vi "Oxford-VRM-v2-Main.vi"() -> ()   [LabVIEW 2016]
uses:
  <instrlib>/Mercury iXX/Public/Libraries/Magnet/Controls/Device (Read).ctl
  <instrlib>/Mercury iXX/Public/Controls/Manufacturing Data.ctl
  <instrlib>/Mercury iXX/Public/Libraries/Magnet/Controls/Signals (Read).ctl
  <instrlib>/Mercury iXX/Public/Controls/Unit String.ctl
  <instrlib>/Mercury iXX/Public/Libraries/Magnet/Controls/Identifier.ctl
  <instrlib>/Mercury iXX/Public/Libraries/Magnet/Controls/PSU Actions.ctl
  <instrlib>/Mercury iXX/Public/Controls/Mercury Reference.ctl
  <instrlib>/Mercury iXX/Public/Controls/Comms Transport Layer.ctl
  <instrlib>/Mercury iXX/Private/Controls/Query Dynamic Reference.ctl
  <vilib>/Analysis/coordinate.llb/3D Coordinate Conversion (Scalar).vi
  <instrlib>/Mercury iXX/Public/Libraries/Magnet/Open/Open Magnet Device.vi
  <instrlib>/Mercury iXX/Public/Libraries/Magnet/Configuration/Set/PSU Action Status (Set).vi
  <instrlib>/Mercury iXX/Public/Libraries/Magnet/Signals/Set/Target Field (Set).vi
  <instrlib>/Mercury iXX/Public/Libraries/Magnet/Signals/Set/Target Field Rate (Set).vi
  <userlib>/_OpenG.lib/error/error.llb/Filter Error Codes (Array)__ogtk.vi
  <instrlib>/Mercury iXX/Public/Libraries/System/Open/Open System.vi
  <instrlib>/Mercury iXX/Public/Libraries/System/Read/Catalogue (Read).vi
  <instrlib>/Mercury iXX/Public/Libraries/System/Read/Display Automatic Dimming (Read).vi
  <instrlib>/Mercury iXX/Public/Libraries/System/Read/Display Automatic Dimming Time (Read).vi
  <instrlib>/Mercury iXX/Public/Libraries/System/Read/Display Brightness (Read).vi
  <instrlib>/Mercury iXX/Public/Libraries/System/Read/Date (Read).vi
  <instrlib>/Mercury iXX/Public/Libraries/System/Read/Time (Read).vi
  <instrlib>/Mercury iXX/Public/Libraries/System/Read/DateTime (Read).vi
  <instrlib>/Mercury iXX/Public/Libraries/System/Read/HVer (Read).vi
  <instrlib>/Mercury iXX/Public/Libraries/System/Read/FVer (Read).vi
  <instrlib>/Mercury iXX/Public/Libraries/System/Read/Serial Number (Read).vi
  <instrlib>/Mercury iXX/Public/Libraries/System/Read/Flash Space (Read).vi
  <instrlib>/Mercury iXX/Public/Libraries/System/Read/Mode (Read).vi
  <instrlib>/Mercury iXX/Public/Libraries/System/Set/DateTime (Set).vi
  <instrlib>/Mercury iXX/Public/Libraries/Magnet/Configuration/Read/Magnet Device (Read).vi
  <instrlib>/Mercury iXX/Public/Libraries/Magnet/Configuration/Read/Serial Number (Read).vi
  <instrlib>/Mercury iXX/Public/Libraries/Magnet/Configuration/Read/Bipolar Output (Read).vi
  <instrlib>/Mercury iXX/Public/Libraries/Magnet/Configuration/Read/Output Configuration (Read).vi
  <instrlib>/Mercury iXX/Public/Libraries/Magnet/Configuration/Read/Current Limit (Read).vi
  <instrlib>/Mercury iXX/Public/Libraries/Magnet/Configuration/Read/Current to Field Factor (Read).vi
  <instrlib>/Mercury iXX/Public/Libraries/Magnet/Configuration/Read/Switch Present (Read).vi
  <instrlib>/Mercury iXX/Public/Libraries/Magnet/Configuration/Read/Software Voltage Limit (Read).vi
  <instrlib>/Mercury iXX/Public/Libraries/Magnet/Signals/Read/Current Rate (Read).vi
  <instrlib>/Mercury iXX/Public/Libraries/Magnet/Configuration/Read/PSU Action Status (Read).vi
  <instrlib>/Mercury iXX/Public/Libraries/Magnet/Signals/Read/Target Field (Read).vi
  <instrlib>/Mercury iXX/Public/Libraries/Magnet/Signals/Read/Field (Read).vi
  <instrlib>/Mercury iXX/Public/Libraries/Magnet/Signals/Read/Target Field Rate (Read).vi
  <instrlib>/Mercury iXX/Public/Libraries/Magnet/Signals/Read/Current (Read).vi
  <instrlib>/Mercury iXX/Public/Libraries/Magnet/Signals/Read/Voltage (Read).vi
  <instrlib>/Mercury iXX/Public/Libraries/Magnet/Configuration/Read/FVer (Read).vi
  <instrlib>/Mercury iXX/Mercury iXX.lvlib
  <instrlib>/Mercury iXX/Public/Libraries/System.lvlib
  <instrlib>/Mercury iXX/Public/Libraries/Magnet.lvlib
  <vilib>/Analysis/NI_AALPro.lvlib
panel:
  out "Firmware Version 2":string
  in  "Device Identifier 2":T1="GRPZ"
  in  "Tab Control":T2(tab)
  out "Z Magnet Status":string="Holding"
  out "Y Magnet Status":string="Holding"
  in  "Tab Control 3":enum32{"Main", "Zero/Clamp"}(tab)
  out "Time (min)":dbl
  in  "OK":bool
  in  "Remote Mode":bool
  in  "Hold":bool
  in  "To Set":bool
  in  "Send to IPS":bool
  in  "Sweep Rate (T/min)":dbl
  in  "Clamp":bool
  in  "To Zero":bool
  in  "Tab Control 2":enum32{"Cartesian", "Spherical"}(tab)
  in  "X Setpoint (T)":dbl
  in  "Y Setpoint (T)":dbl
  in  "Z Setpoint (T)":dbl
  out "X Target (T)":dbl
  out "X Field (T)":dbl=-0.0
  out "Y Target (T)":dbl
  out "Y Field (T)":dbl
  out "Z Target (T)":dbl
  out "Z Field (T)":dbl
  in  "R Setpoint (T)":dbl
  in  "Theta Setpoint (deg)":dbl
  in  "Phi Setpoint (deg)":dbl
  out "R Target (T)":dbl
  out "R Field (T)":dbl
  out "Theta Target (deg)":dbl
  out "Theta Field (deg)":dbl=180.0
  out "Phi Target (deg)":dbl
  out "Phi Field (deg)":dbl
  out "Sentinel":bool=TRUE
  out "Z Voltage (V)":dbl=-0.0001
  out "Z Current (A)":dbl
  out "Z Rate (T/min)":dbl=0.05
  out "Y Voltage (V)":dbl
  out "Y Current (A)":dbl=0.0001
  out "Y Rate (T/min)":dbl=0.0002
  out "X Voltage (V)":dbl=0.0003
  out "X Current (A)":dbl=-0.0001
  out "X Rate (T/min)":dbl=0.0002
  out "Magnet Response":string
  out "X Magnet Status":string="Holding"
  in  "Tab Control 4":enum32{"Graph", "Limits", "Definitions"}(tab)
  out "3D Graph":refnum<vi>(3d-picture)
  out "Legend":refnum<vi>(3d-picture)
  in  "Mercury Functions":enum32{"System: IPS", "Magnet"}(tab)
  out "time stamp":timestamp=timestamp(3548852719 s since 1904-01-01)
  out "Free Space 2":i32=167300 caption="Free Space (KB)"
  out "Set Date Response":string="VALID"
  out "String 2":string="NORM" caption="User Mode"
  out "Date":string="2016:06:15"
  out "Time":string="11:26:27"
  out "Hardware Version":string="65"
  out "Firmware Version":string="1.4.43"
  out "Serial Number":string="133350022"
  out "IPS Devices":string[](array[string])=["GRPX:PSU", "GRPY:PSU", "GRPZ:PSU", "MB1.T1:TEMP", "PSU.M1:PSU", "PSU.M2:PSU", "PSU.M3:PSU", "PSU.M4:PSU", "PSU.M5:PSU", "PSU.M6:PSU"]
  out "S/W Version(s)":string[](array[string])=["1.4.43\n"]
  out "Serial Number(s)":string[](array[string])=["65"]
  out "# of Instruments":i32=1
  out "Automatic Dimming":string="OFF"
  out "Dimming Time":string="3"
  out "Display Brightness":string="100"
  in  "IPS IP Address":string="130.49.180.67"
  out "Magnet Device Details":T3={"Manufacturing"={"Hardware Version"="NOT_FOUND", "Firmware Version"="NOT_FOUND", "Serial Number"="NOT_FOUND"}, "Nickname"="GRPX", "Bipolar Output"="ON", "String"="PARA", "Current Limit"=99.07, "AtoB"=49.5, "Inductance"=5.04, "Switch Present"="None", "Swh Htr Current"=100.0, "SW VLIM"=5.0, "V Trans Time"=0.0, "Magnet PSU Signals"={"Voltage"=0.0007, "Current"=0.0001, "Current Rate"=0.01, "Field"=0.0, "Field Rate"=0.0002, "Persistant Current"=0.0001, "Persistant Field"=0.0, "Target Current"=0.0, "Target Field"=0.0, "Target Current Rate"=0.01, "Target Field Rate"=0.0002, "Switch Heater Status (SWHT)"="ON", "Switch Heater Status (SWHN)"="ON"}, "PSU Action"="HOLD", "Status"="40000000", "Level Limit"=0.0, "Temperature Limit"=999.0} {"Temperature Limit" format="%#.1f"; "Level Limit" format="%#.1f"; "V Trans Time" format="%#.1f"; "SW VLIM" format="%#.1f"; "Swh Htr Current" format="%#.1f"; "Inductance" format="%#.1f"; "AtoB" format="%#.1f"; "Current Limit" format="%#.1f"}
  out "Mag S/N":string="NOT_FOUND"
  out "Bipolar Output":string="ON"
  out "Out Config":string="PARA" caption="Output Configuration"
  out "Current Limit":dbl=99.07 caption="Current Limit (A)" format="%#.1f"
  out "AtoB":dbl=49.5 caption="Current Field Factor (A/T)" format="%#.1f"
  out "Switch Present":string="None"
  out "SW VLIM":dbl=5.0 caption="Software Voltage Limit (V)" format="%#.1f"
  out "Unit 8":T6
  out "Unit 9":T6
  out "Unit 10":T6
  out "Current Rate":dbl=0.01
  out "PSU Act Stat":string="HOLD" caption="PSU Action Status"
  out "Unit 11":T6="A/min"
  in  "Device Identifier":T1="GRPX"
  out "Error List":T7(array[cluster])=[{"time"=timestamp(3548847490.5163774 s since 1904-01-01), "code"=-1950679035, "source"="Open Variable Connection in FGV_PSP - Mercury Remote.vi->Mercury iXX.lvlib:Oxford-VRM-v2-Main.vi"}, {"time"=timestamp(3548847496.0233774 s since 1904-01-01), "code"=-1950679035, "source"="Open Variable Connection in FGV_PSP - Mercury Remote.vi->Mercury iXX.lvlib:Oxford-VRM-v2-Main.vi"}, {"time"=timestamp(3548847520.519377 s since 1904-01-01), "code"=-1950679035, "source"="Open Variable Connection in FGV_PSP - Mercury Status.vi->Mercury iXX.lvlib:Oxford-VRM-v2-Main.vi"}, {"time"=timestamp(3548847557.480377 s since 1904-01-01), "code"=-1950679035, "source"="Open Variable Connection in FGV_PSP - Mercury Remote.vi->Mercury iXX.lvlib:Oxford-VRM-v2-Main.vi"}, {"time"=timestamp(3548847576.0283775 s since 1904-01-01), "code"=-1950679035, "source"="Open Variable Connection in FGV_PSP - Mercury Status.vi->Mercury iXX.lvlib:Oxford-VRM-v2-Main.vi"}]
  out "error out":errorcluster
  # "Oxford VRM v2 v2016/06/22"
  # "X \t\t\nCurrent (A)\tField (T)\t    Rate (T/min)\n0  - 30 \t   0    - 0.6 \t  0.06\n30 - 42\t    0.6  - 0.85\t  0.048\n42 - 60\t    0.85 - 1.2\t   0.042\n60 - 80\t    1.2  - 1.6\t   0.036\n80 - 99\t    1.6  - 2.0\t   0.024\n\nY \t\t\nCurrent (A)\tField (T)\t    Rate (T/min)\n0  - 30\t    0    - 0.6\t   0.048\n30 - 35\t    0.6  - 0.69\t  0.035\n35 - 45\t    0.69 - 0.89\t  0.03\n45 - 60\t    0.89 - 1.2\t   0.024\n60 - 80\t    1.2  - 1.58\t  0.018\n80 - 101\t   1.58 - 2\t     0.01\n\nZ \t\t\nCurrent (A)\tField (T)\t    Rate (T/min)\n0  - 30\t    0    - 2.6    0.26\n30 - 60\t    2.6  - 5.3\t   0.21\n60 - 80\t    5.3  - 7.1\t   0.16\n80 - 90\t    7.1  - 8\t     0.13\n90 - 101\t   8    - 9\t     0.1\n\n2 OR MORE AXES\n0.005 T/min"
  # "ITC: 101\nIPS: 102\nIPS VR: 67"
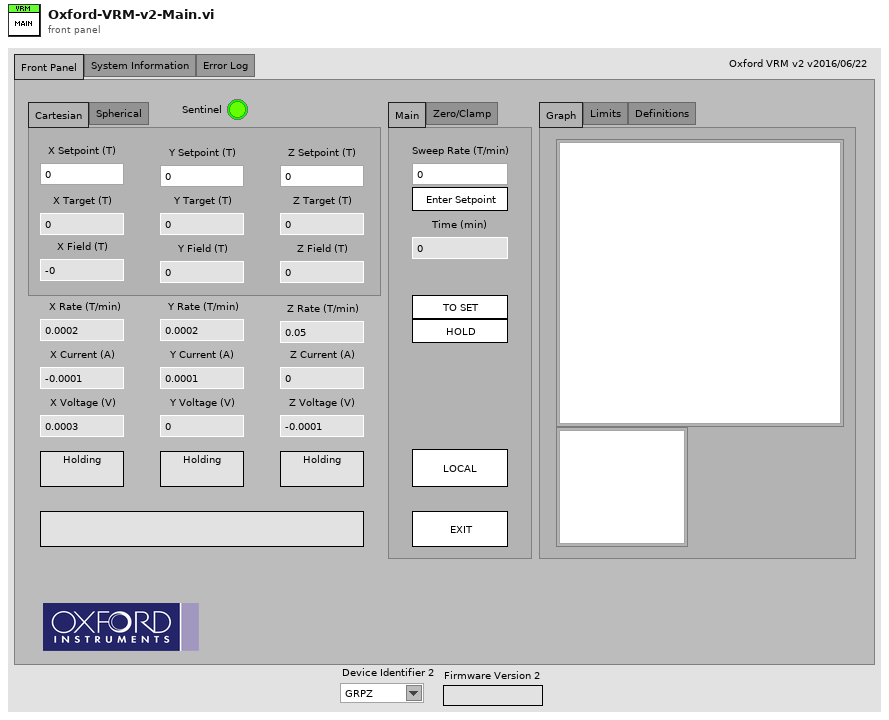
[diagram p1: front panel]
types:
  T1 = typedef "Mercury iXX.lvlib/Magnet.lvlib/Identifier.ctl" = string
  T2 = enum32{"Front Panel", "System Information", "Error Log"}
  T3 = typedef "Mercury iXX.lvlib/Magnet.lvlib/Device (Read).ctl" = cluster{"Manufacturing":T4, "Nickname":string, "Bipolar Output":string, "String":string, "Current Limit":dbl, "AtoB":dbl, "Inductance":dbl, "Switch Present":string, "Swh Htr Current":dbl, "SW VLIM":dbl, "V Trans Time":dbl, "Magnet PSU Signals":T5, "PSU Action":string, "Status":string, "Level Limit":dbl, "Temperature Limit":dbl}
  T4 = typedef "Mercury iXX.lvlib/Manufacturing Data.ctl" = cluster{"Hardware Version":string, "Firmware Version":string, "Serial Number":string}
  T5 = typedef "Mercury iXX.lvlib/Magnet.lvlib/Signals (Read).ctl" = cluster{"Voltage":dbl, "Current":dbl, "Current Rate":dbl, "Field":dbl, "Field Rate":dbl, "Persistant Current":dbl, "Persistant Field":dbl, "Target Current":dbl, "Target Field":dbl, "Target Current Rate":dbl, "Target Field Rate":dbl, "Switch Heater Status (SWHT)":string, "Switch Heater Status (SWHN)":string}
  T6 = typedef "Mercury iXX.lvlib/Unit String.ctl" = string
  T7 = cluster{"time":timestamp, "code":i32, "source":string}[]
  T8 = cluster{"Hold":bool, "Clamp":bool, "To Set":bool, "To Zero":bool, "Send to IPS":bool}
  T9 = cluster{"Bx0 (T)":dbl, "By0 (T)":dbl, "Bz0 (T)":dbl}
  T10 = cluster{"Bx (T)":dbl, "By (T)":dbl, "Bz (T)":dbl}
  T11 = enum32{"invalid app kind", "Development System", "Run Time System", "Student Edition", "Embedded LabVIEW", "Evaluation", "Custom"}
  T12 = cluster{"time":timestamp, "code":i32, "source":string}
  T13 = enum32{"Invalid", "Standard", "Closed", "Hidden", "Minimized", "Maximized"}
  T14 = typedef "Mercury iXX.lvlib/Comms Transport Layer.ctl" = enum16{"Ethernet TCP/IP", "USB", "ISOBus - RS-232", "GPIB"}
  T15 = cluster{"x action":string, "y action":string, "z action":string}
  T16 = typedef "Mercury iXX.lvlib/Mercury Reference.ctl" = cluster{"Comms":refnum<visa-resource-name>, "Device ID":string[], "Comms Layer":T14, "Command":string, "Query reference":T17}
  T17 = typedef "Mercury iXX.lvlib/Query Dynamic Reference.ctl" = refnum<vi>
  T18 = cluster{"Core":cluster{"Current VI Reference":refnum<vi>, "Close Panel on Exit?":bool}, "Mercury IPS Ref":T16, "sentinel":bool, "Error Log":cluster{"time":timestamp, "code":i32, "source":string}[]}
  T19 = cluster{"X Setpoint (T)":dbl, "Y Setpoint (T)":dbl, "Z Setpoint (T)":dbl, "Sweep Rate (T/min)":dbl}
  T20 = typedef "Mercury iXX.lvlib/Magnet.lvlib/PSU Actions.ctl" = string
  T21 = typedef "Mercury iXX.lvlib/Response String.ctl" = string
  T22 = cluster{"Rate_x (T/min)":dbl, "Rate_y (T/min)":dbl, "Rate_z (Tmin)":dbl}
  T23 = typedef "Filtered Error Details - Cluster__ogtk.ctl" = cluster{"code":i32, "source":string}
  T24 = cluster{"Current VI Reference":refnum<vi>, "Close Panel on Exit?":bool}
  T25 = typedef "Mercury iXX.lvlib/System.lvlib/User Mode.ctl" = string
  T26 = typedef "Mercury iXX.lvlib/Magnet.lvlib/Output Configuration.ctl" = string
  T27 = cluster{"X Target (T)":dbl, "Y Target (T)":dbl, "Z Target (T)":dbl, "X Field (T)":dbl, "Y Field (T)":dbl, "Z Field (T)":dbl, "X Rate (T/min)":dbl, "Y Rate (T/min)":dbl, "Z Rate (T/min)":dbl, "X Current (A)":dbl, "Y Current (A)":dbl, "Z Current (A)":dbl, "X Voltage (V)":dbl, "Y Voltage (V)":dbl, "Z Voltage (V)":dbl}
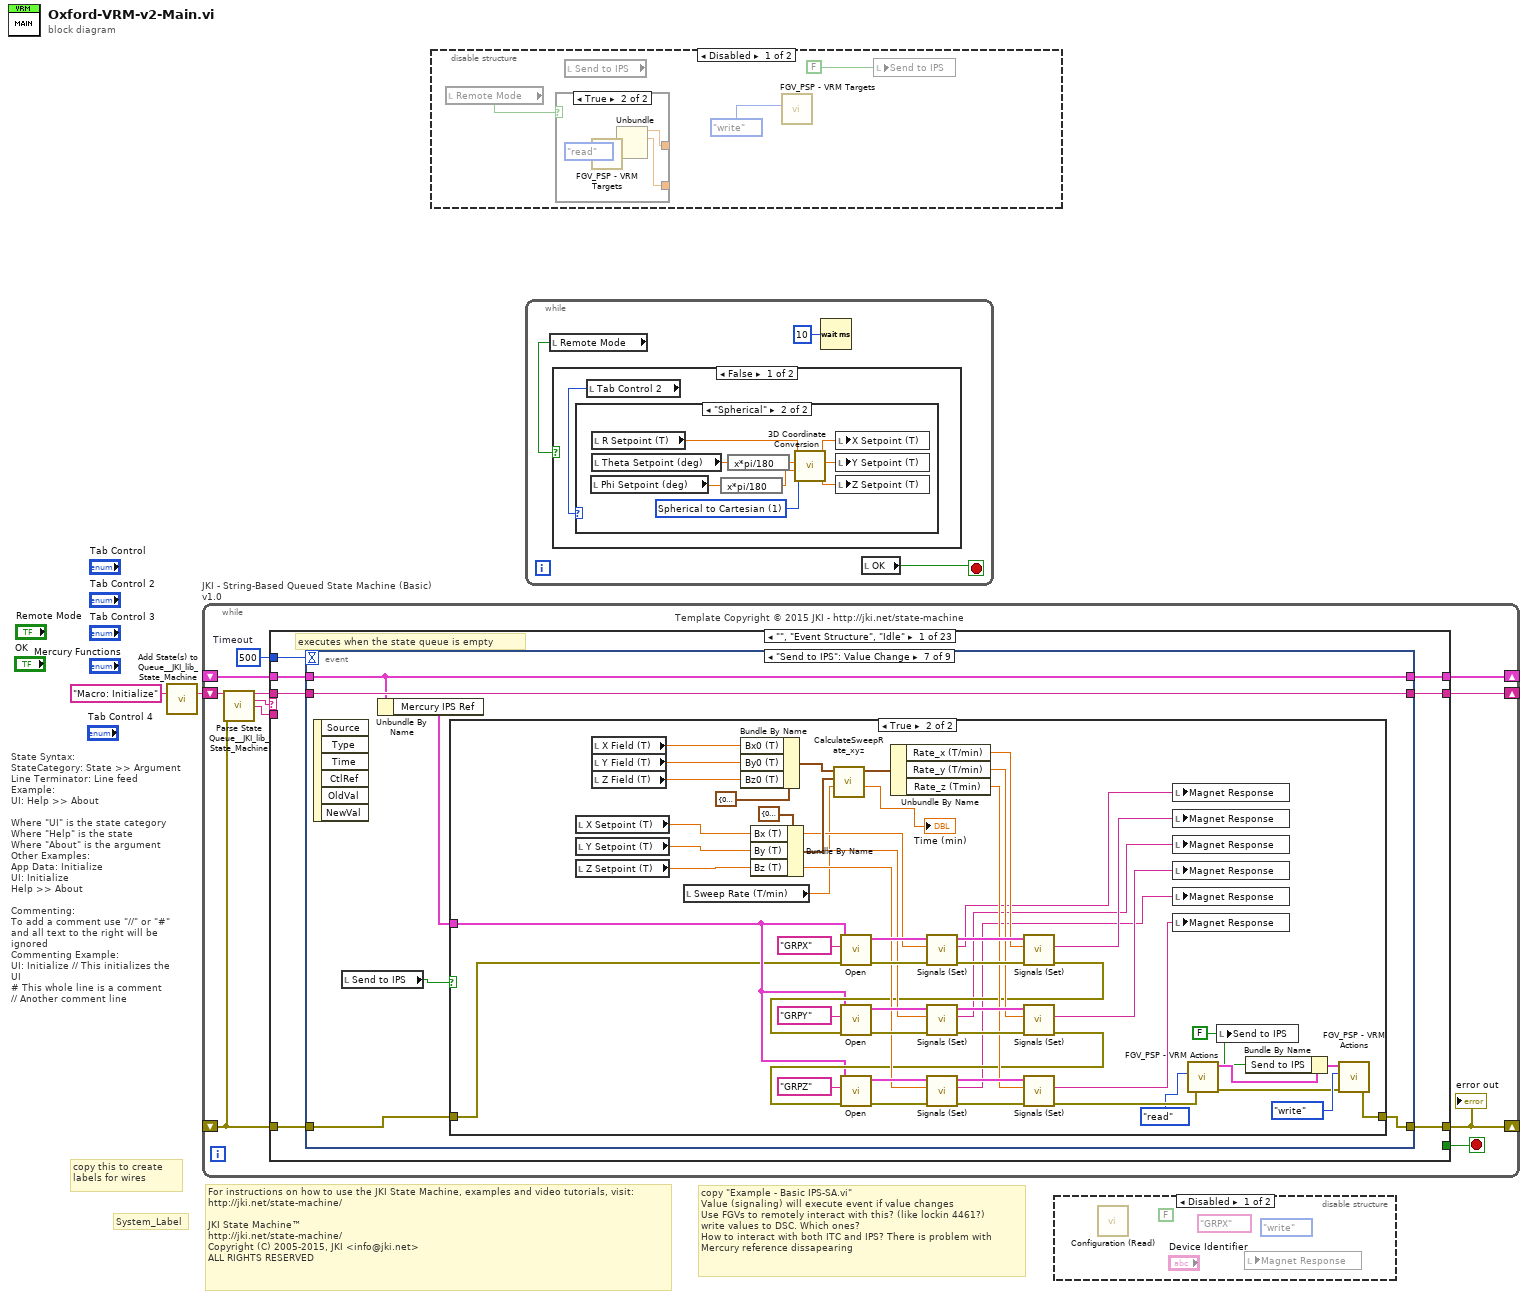
[diagram p0: block diagram]
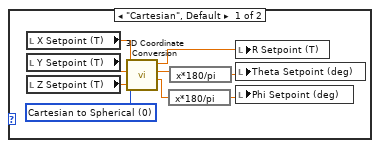
[diagram p2: hidden frame]
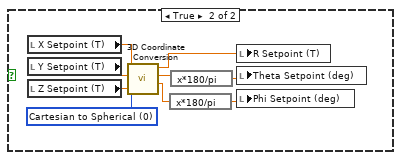
[diagram p3: hidden frame]
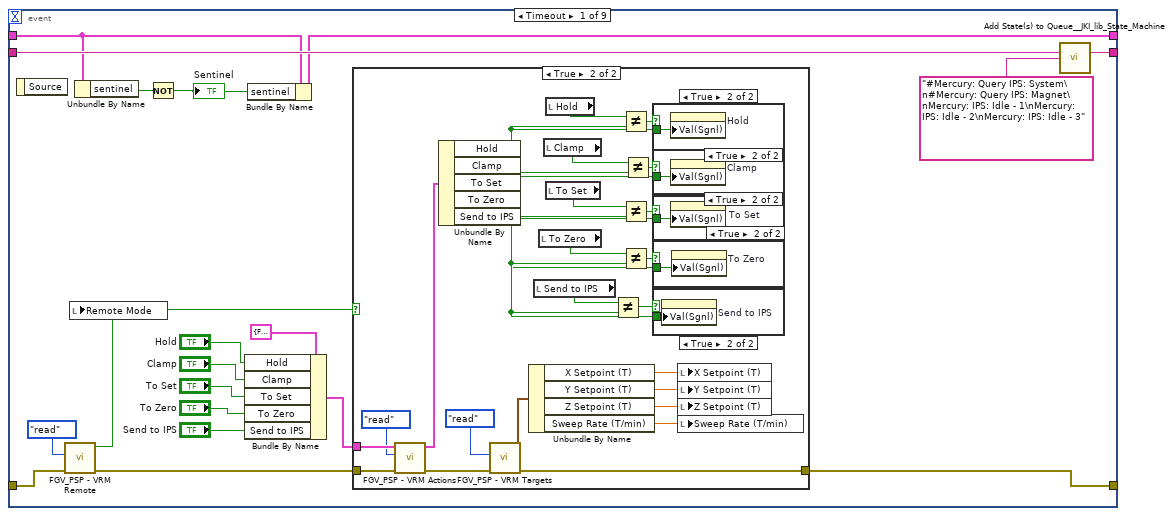
[diagram p7: hidden frame]
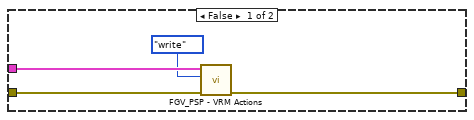
[diagram p8: hidden frame]
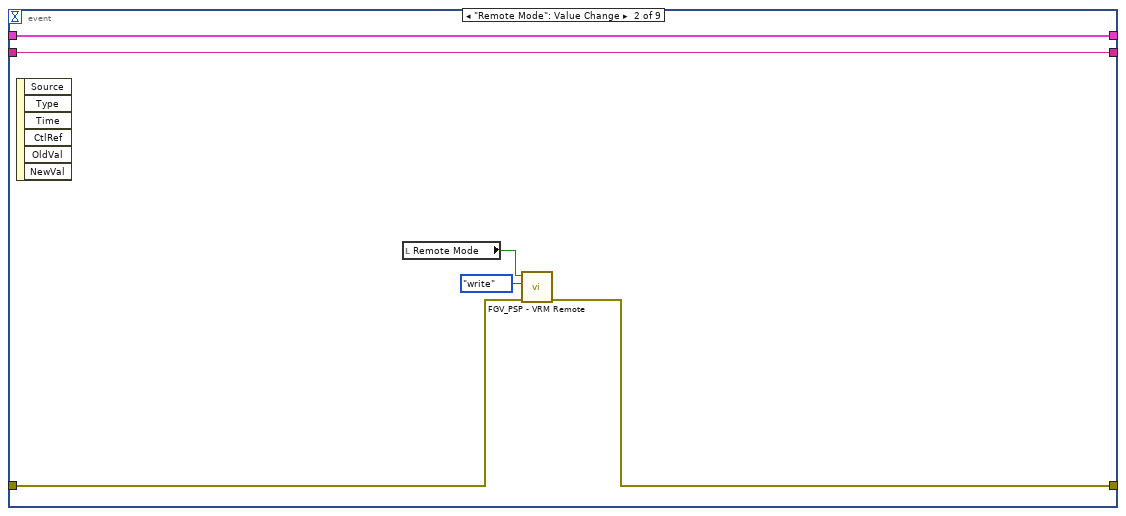
[diagram p14: hidden frame]
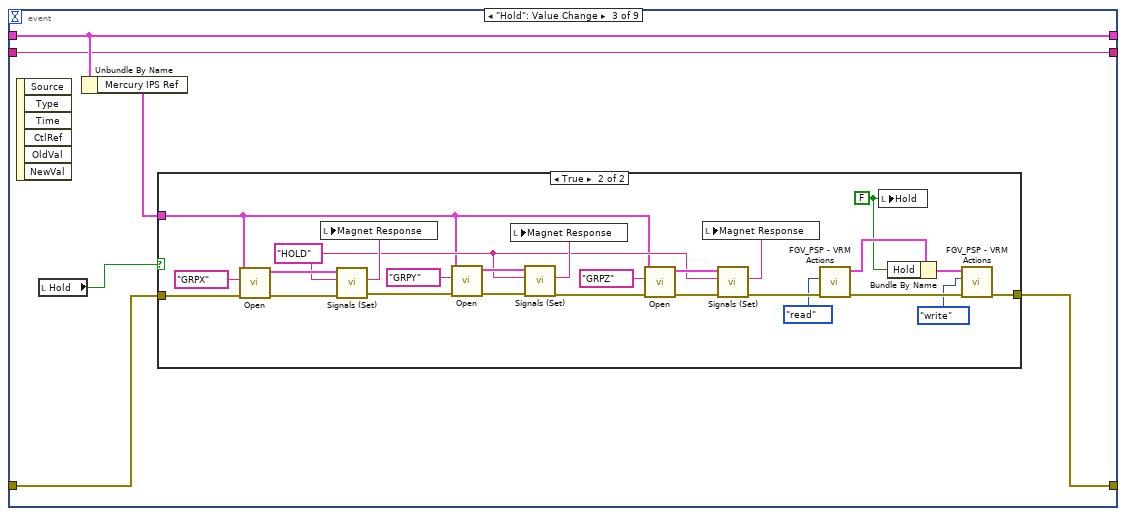
[diagram p15: hidden frame]
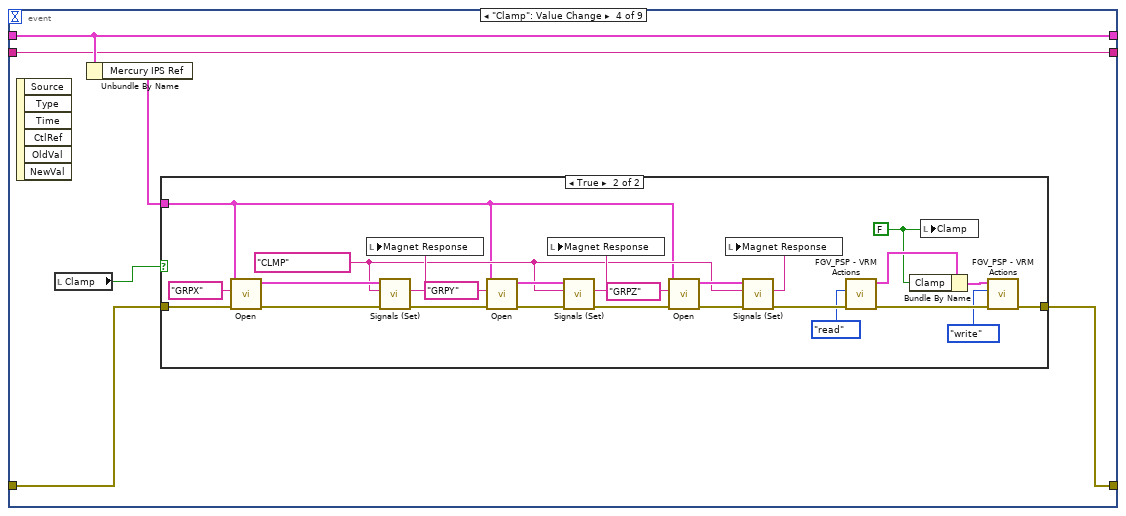
[diagram p17: hidden frame]
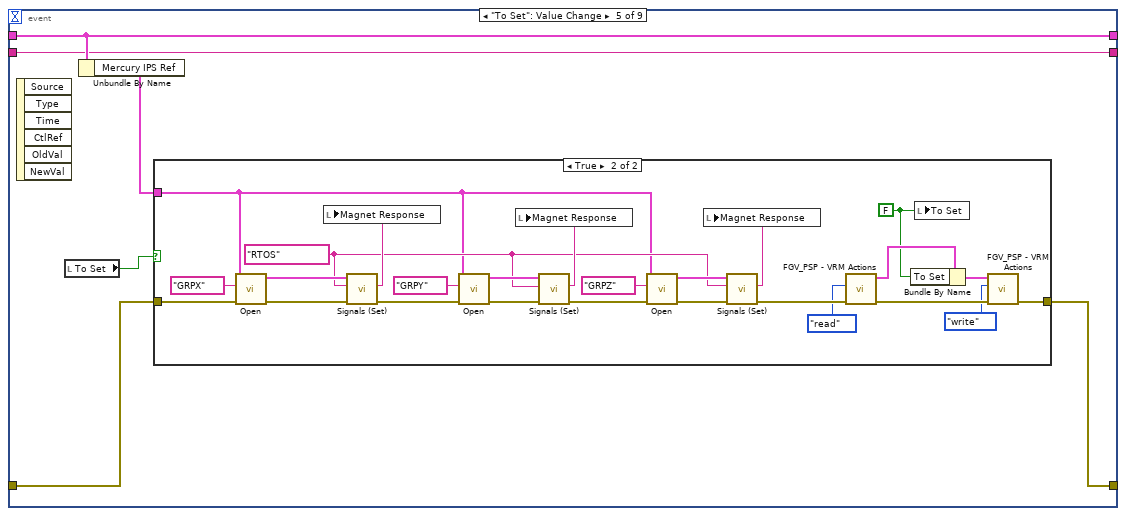
[diagram p19: hidden frame]
diagram:
  # "copy \"Example - Basic IPS-SA.vi\"\nValue (signaling) will execute event if value changes\nUse FGVs to remotely interact with this? (like lockin 4461?)\nwrite values to DSC. Which ones?\nHow to interact with both ITC and IPS? There is problem with \nMercury reference dissapearing"
  # "For instructions on how to use the JKI State Machine, examples and video tutorials, visit:\nhttp://jki.net/state-machine/\n\nJKI State Machine™\nhttp://jki.net/state-machine/\nCopyright (C) 2005-2015, JKI <info@jki.net>\nALL RIGHTS RESERVED"
  # "State Syntax:\nStateCategory: State >> Argument\nLine Terminator: Line feed\nExample:\nUI: Help >> About\n\nWhere \"UI\" is the state category\nWhere \"Help\" is the state\nWhere \"About\" is the argument\nOther Examples:\nApp Data: Initialize\nUI: Initialize\nHelp >> About\n\nCommenting:\nTo add a comment use \"//\" or \"#\" and all text to the right will be ignored\nCommenting Example:\nUI: Initialize // This initializes the UI\n# This whole line is a comment\n// Another comment line"
  # "copy this to create labels for wires"
  # "System_Label"
  n1 = call <vilib>:"Add State(s) to Queue__JKI_lib_State_Machine.vi"("State(s) in (\"\")"="Macro: Initialize") -> ("States Out"=w2:string)  [unwired: 14 in]
  n2 = while "JKI - String-Based Queued State Machine (Basic) v1.0" {
    shift-right: [w7] -> _
    shift-left: _ -> [w6]
    shift-right: [w3] -> _
    shift-left: _ -> [w4]
    shift-right: [w9] -> _
    shift-left: w2 -> [w10]
    stop <- w8 stop-if-true
    w5 = 500  # Timeout
    # "Template Copyright © 2015 JKI - http://jki.net/state-machine"
    n3 = call <vilib>:"Parse State Queue__JKI_lib_State_Machine.vi"("State Queue"=w10, "Error In (no error)"=w4) -> ("Remaining States"=w12:string, "Current State"=w13:string, "Arguments"=w11:string)  [unwired: 11 in]
    n4 = case shown="\"\", \"Event Structure\", \"Idle\"" w13 {
      selector: w13 -> [_ _ w279 _ _ _ _ _ _ _ _ _ _ _ _ _ _ _ _ _ _ _ _]
      tunnel: w12 -> [w20 w278 w283 w301 w318 w323 w327 w335 w341 w345 w369 w382 w393 w419 w424 w450 w454 w469 w513 w553 w634 w659 w668]
      tunnel: w11 -> [_ _ _ _ _ _ _ _ _ _ _ w377 w387 _ _ _ _ _ _ _ _ _ _]
      tunnel: w6 -> [w16 w275 w281 w292 w304 w321 w324 _ w336 w342 w367 w380 w389 w416 w422 w448 w451 w467 w511 w552 w633 w658 w667]
      tunnel: [w14 w276 w285 w298 errorcluster {"status"=FALSE, "code"=0, "source"=""} ("error out") w320 w325 w329 w337 w343 w354 w378 w390 w417 w421 w433 w452 w458 w475 w519 w556 w644 w666] -> w3
      tunnel: [w19 w277 w282 w300 w317 w322 w326 w334 w340 w344 w368 w381 w392 w418 w423 w449 w453 w468 w512 w554 w635 w660 w669] -> w9
      tunnel: [_ _ _ _ _ TRUE _ _ _ _ _ _ _ _ _ _ _ _ _ _ _ _ _] -> w8
      tunnel: [w18 w275 w281 w299 w303 w321 w324 w333 w336 w342 w367 w380 w389 w416 w422 w448 w451 w466 w511 w552 w633 w658 w667] -> w7
      tunnel: w5 -> [w17 _ _ _ _ _ _ _ _ _ _ _ _ _ _ _ _ _ _ _ _ _ _]
      tunnel: w4 -> [w15 w276 w284 w298 w313 w320 w325 w329 w338 w343 w355 w379 w391 w417 w421 w441 w452 w455 w477 w515 w632 w645 w666]
      frame "", "Event Structure", "Idle" {
        # "executes when the state queue is empty"
        n5 = event shown="[6] \"Send to IPS\": Value Change" {
          selector: _ -> [_ _ _ _ _ _ _ _ _]
          dyn-events: _ -> [_ _ _ _ _ _ _ _ _]
          timeout: w17 -> [_ _ _ _ _ _ _ _ _]
          tunnel: w20 -> [w39 w78 w86 w118 w150 w183 w213 w268 w274]
          tunnel: [w38 w78 w86 w118 w150 w183 w213 w267 w273] -> w19
          tunnel: [w33 w77 w87 w119 w151 w182 w212 w265 w271] -> w18
          tunnel: w16 -> [w34 w77 w87 w119 w151 w182 w212 w265 w271]
          tunnel: w15 -> [w25 w80 w84 w116 w148 w180 w209 w266 w272]
          tunnel: [w22 w79 w85 w117 w149 w181 w210 w266 w272] -> w14
          event Timeout {
            n6 = event-data() -> ()  [unwired: 1 in, 1 out]
            n7 = call "FGV_PSP - VRM Remote.vi"("error in"=w25, "Function"=enum16{"write", "read"}."read") -> ("error out"=w24:errorcluster, "VRM Remote"=w21:bool)  [unwired: 4 in]
            n8 = local write "Remote Mode"(w21) -> ()
            n9 = Unbundle By Name(w34) -> ("sentinel"=w36:bool)
            n10 = Not(x=w36) -> (.not. x?=w35:bool)
            "Sentinel" <- w35
            n11 = Bundle By Name(cluster=T8 {"Hold"=FALSE, "Clamp"=FALSE, "To Set"=FALSE, "To Zero"=FALSE, "Send to IPS"=FALSE}, "Hold"="Hold", "Clamp"="Clamp", "To Set"="To Set", "To Zero"="To Zero", "Send to IPS"="Send to IPS") -> (w29:T8)
            n12 = Bundle By Name(cluster=w34, "sentinel"=w35) -> (w33:T18)
            n13 = case shown="True" w21 {
              tunnel: [w42 w52] -> w22
              tunnel: w24 -> [w43 w70]
              tunnel: w29 -> [w41 w69]
              frame False {
                n14 = call "FGV_PSP - VRM Actions.vi"("error in"=w43, "Function"=enum16{"write", "read"}."write", "VRM actions"=w41) -> ("error out"=w42:errorcluster)  [unwired: 3 in, 1 out]
              }
              frame True {
                n15 = call "FGV_PSP - VRM Actions.vi"("error in"=w70, "Function"=enum16{"write", "read"}."read", "VRM actions"=w69) -> ("error out"=w53:errorcluster, "VRM actions"=w44:T8)  [unwired: 3 in]
                n16 = Unbundle By Name(w44) -> ("Hold"=w59:bool, "Clamp"=w47:bool, "To Set"=w61:bool, "To Zero"=w62:bool, "Send to IPS"=w63:bool)
                n17 = call "FGV_PSP - VRM Targets.vi"("error in"=w53, "Function"=enum16{"write", "read"}."read") -> ("error out"=w52:errorcluster, "VRM Targets 2"=w46:T19)  [unwired: 4 in]
                n18 = Unbundle By Name(w46) -> ("X Setpoint (T)"=w51:dbl, "Y Setpoint (T)"=w50:dbl, "Z Setpoint (T)"=w49:dbl, "Sweep Rate (T/min)"=w48:dbl)
                n19 = local read "Send to IPS"() -> (w60:bool)
                n20 = local read "To Zero"() -> (w58:bool)
                n21 = local read "Clamp"() -> (w56:bool)
                n22 = local read "Hold"() -> (w55:bool)
                n23 = local read "To Set"() -> (w57:bool)
                n24 = Not Equal?(x=w60, y=w63) -> (x != y?=w64:bool)
                n25 = Not Equal?(x=w55, y=w59) -> (x != y?=w68:bool)
                n26 = Not Equal?(x=w57, y=w61) -> (x != y?=w66:bool)
                n27 = Not Equal?(x=w58, y=w62) -> (x != y?=w65:bool)
                n28 = Not Equal?(x=w56, y=w47) -> (x != y?=w67:bool)
                n29 = case shown="True" w68 {
                  tunnel: w59 -> [_ w75]
                  frame False {
                  }
                  frame True {
                    n30 = property on="Hold" class="Bool (strict)"("Val(Sgnl)"=w75) -> ()  [unwired: 2 in, 2 out]
                  }
                }
                n31 = case shown="True" w67 {
                  tunnel: w47 -> [_ w74]
                  frame False {
                  }
                  frame True {
                    n32 = property on="Clamp" class="Bool (strict)"("Val(Sgnl)"=w74) -> ()  [unwired: 2 in, 2 out]
                  }
                }
                n33 = case shown="True" w66 {
                  tunnel: w61 -> [_ w73]
                  frame False {
                  }
                  frame True {
                    n34 = property on="To Set" class="Bool (strict)"("Val(Sgnl)"=w73) -> ()  [unwired: 2 in, 2 out]
                  }
                }
                n35 = case shown="True" w65 {
                  tunnel: w62 -> [_ w72]
                  frame False {
                  }
                  frame True {
                    n36 = property on="To Zero" class="Bool (strict)"("Val(Sgnl)"=w72) -> ()  [unwired: 2 in, 2 out]
                  }
                }
                n37 = case shown="True" w64 {
                  tunnel: w63 -> [_ w71]
                  frame False {
                  }
                  frame True {
                    n38 = property on="Send to IPS" class="Bool (strict)"("Val(Sgnl)"=w71) -> ()  [unwired: 2 in, 2 out]
                  }
                }
                n39 = local write "X Setpoint (T)"(w51) -> ()
                n40 = local write "Y Setpoint (T)"(w50) -> ()
                n41 = local write "Z Setpoint (T)"(w49) -> ()
                n42 = local write "Sweep Rate (T/min)"(w48) -> ()
              }
            }
            n43 = call <vilib>:"Add State(s) to Queue__JKI_lib_State_Machine.vi"("State(s) in (\"\")"=w39, "State(s) at Back (\"\")"="#Mercury: Query IPS: System\n#Mercury: Query IPS: Magnet\nMercury: IPS: Idle - 1\nMercury: IPS: Idle - 2\nMercury: IPS: Idle - 3" ("State(s) at Back (\"\")")) -> ("States Out"=w38:string)  [unwired: 13 in]
          }
          event "Remote Mode": Value Change {
            n44 = event-data() -> ()  [unwired: 1 in, 6 out]
            n45 = local read "Remote Mode"() -> (w76:bool)
            n46 = call "FGV_PSP - VRM Remote.vi"("error in"=w80, "Function"=enum16{"write", "read"}."write", "VRM Remote"=w76) -> ("error out"=w79:errorcluster)  [unwired: 3 in, 1 out]
          }
          event "Hold": Value Change {
            n47 = event-data() -> ()  [unwired: 1 in, 6 out]
            n48 = local read "Hold"() -> (w82:bool)
            n49 = Unbundle By Name(w87) -> ("Mercury IPS Ref"=w83:T16)
            n50 = case shown="True" w82 {
              tunnel: [w88 w107] -> w85
              tunnel: w84 -> [w88 w105]
              tunnel: w83 -> [_ w89]
              frame False {
              }
              frame True {
                w110 = FALSE ("Hold")
                w93 = T20 "HOLD" ("PSU Act Stat")
                n51 = call-poly <instrlib>:"Open.vi"("error in (no error)"=w105, "Device Identifier"=T1 "GRPX", "Mercury Reference In"=w89) -> ("error out"=w113:errorcluster, "Mercury Reference Out"=w112:T16)  [unwired: 7 out]
                n52 = call-poly <instrlib>:"Signals (Set).vi"("error in"=w113, "PSU Act Stat"=w93, "Mercury Reference In"=w112) -> ("error out"=w102:errorcluster, "Response"=w94:T21)  [unwired: 1 in, 6 out]
                n53 = local write "Magnet Response"(w94) -> ()
                n54 = call-poly <instrlib>:"Open.vi"("error in (no error)"=w102, "Device Identifier"=T1 "GRPY", "Mercury Reference In"=w89) -> ("error out"=w104:errorcluster, "Mercury Reference Out"=w98:T16)  [unwired: 7 out]
                n55 = call-poly <instrlib>:"Signals (Set).vi"("error in"=w104, "PSU Act Stat"=w93, "Mercury Reference In"=w98) -> ("error out"=w101:errorcluster, "Response"=w95:T21)  [unwired: 1 in, 6 out]
                n56 = local write "Magnet Response"(w95) -> ()
                n57 = call-poly <instrlib>:"Open.vi"("error in (no error)"=w101, "Device Identifier"=T1 "GRPZ", "Mercury Reference In"=w89) -> ("error out"=w103:errorcluster, "Mercury Reference Out"=w97:T16)  [unwired: 7 out]
                n58 = call-poly <instrlib>:"Signals (Set).vi"("error in"=w103, "PSU Act Stat"=w93, "Mercury Reference In"=w97) -> ("error out"=w92:errorcluster, "Response"=w96:T21)  [unwired: 1 in, 6 out]
                n59 = local write "Magnet Response"(w96) -> ()
                n60 = call "FGV_PSP - VRM Actions.vi"("error in"=w92, "Function"=enum16{"write", "read"}."read") -> ("error out"=w108:errorcluster, "VRM actions"=w111:T8)  [unwired: 4 in]
                n61 = local write "Hold"(w110) -> ()
                n62 = Bundle By Name(cluster=w111, "Hold"=w110) -> (w109:T8)
                n63 = call "FGV_PSP - VRM Actions.vi"("error in"=w108, "Function"=enum16{"write", "read"}."write", "VRM actions"=w109) -> ("error out"=w107:errorcluster)  [unwired: 3 in, 1 out]
              }
            }
          }
          event "Clamp": Value Change {
            n64 = event-data() -> ()  [unwired: 1 in, 6 out]
            n65 = local read "Clamp"() -> (w114:bool)
            n66 = Unbundle By Name(w119) -> ("Mercury IPS Ref"=w115:T16)
            n67 = case shown="True" w114 {
              tunnel: [w120 w140] -> w117
              tunnel: w116 -> [w120 w138]
              tunnel: w115 -> [_ w121]
              frame False {
              }
              frame True {
                w122 = FALSE
                w126 = T20 "CLMP" ("PSU Act Stat")
                n68 = call-poly <instrlib>:"Open.vi"("error in (no error)"=w138, "Device Identifier"=T1 "GRPX" ("Device Identifier 2"), "Mercury Reference In"=w121) -> ("error out"=w145:errorcluster, "Mercury Reference Out"=w144:T16)  [unwired: 7 out]
                n69 = call-poly <instrlib>:"Signals (Set).vi"("error in"=w145, "PSU Act Stat"=w126, "Mercury Reference In"=w144) -> ("error out"=w131:errorcluster, "Response"=w127:T21)  [unwired: 1 in, 6 out]
                n70 = local write "Magnet Response"(w127) -> ()
                n71 = call-poly <instrlib>:"Open.vi"("error in (no error)"=w131, "Device Identifier"=T1 "GRPY" ("Device Identifier 2"), "Mercury Reference In"=w121) -> ("error out"=w135:errorcluster, "Mercury Reference Out"=w136:T16)  [unwired: 7 out]
                n72 = call-poly <instrlib>:"Signals (Set).vi"("error in"=w135, "PSU Act Stat"=w126, "Mercury Reference In"=w136) -> ("error out"=w130:errorcluster, "Response"=w128:T21)  [unwired: 1 in, 6 out]
                n73 = local write "Magnet Response"(w128) -> ()
                n74 = call-poly <instrlib>:"Open.vi"("error in (no error)"=w130, "Device Identifier"=T1 "GRPZ" ("Device Identifier 2"), "Mercury Reference In"=w121) -> ("error out"=w134:errorcluster, "Mercury Reference Out"=w133:T16)  [unwired: 7 out]
                n75 = call-poly <instrlib>:"Signals (Set).vi"("error in"=w134, "PSU Act Stat"=w126, "Mercury Reference In"=w133) -> ("error out"=w125:errorcluster, "Response"=w129:T21)  [unwired: 1 in, 6 out]
                n76 = local write "Magnet Response"(w129) -> ()
                n77 = call "FGV_PSP - VRM Actions.vi"("error in"=w125, "Function"=enum16{"write", "read"}."read") -> ("error out"=w141:errorcluster, "VRM actions"=w143:T8)  [unwired: 4 in]
                n78 = Bundle By Name(cluster=w143, "Clamp"=w122) -> (w142:T8)
                n79 = local write "Clamp"(w122) -> ()
                n80 = call "FGV_PSP - VRM Actions.vi"("error in"=w141, "Function"=enum16{"write", "read"}."write", "VRM actions"=w142) -> ("error out"=w140:errorcluster)  [unwired: 3 in, 1 out]
              }
            }
          }
          event "To Set": Value Change {
            n81 = event-data() -> ()  [unwired: 1 in, 6 out]
            n82 = local read "To Set"() -> (w146:bool)
            n83 = Unbundle By Name(w151) -> ("Mercury IPS Ref"=w147:T16)
            n84 = case shown="True" w146 {
              tunnel: [w152 w171] -> w149
              tunnel: w148 -> [w152 w168]
              tunnel: w147 -> [_ w155]
              frame False {
              }
              frame True {
                w172 = FALSE
                w157 = T20 "RTOS" ("PSU Act Stat")
                n85 = call-poly <instrlib>:"Open.vi"("error in (no error)"=w168, "Device Identifier"=T1 "GRPX" ("Device Identifier 2"), "Mercury Reference In"=w155) -> ("error out"=w176:errorcluster, "Mercury Reference Out"=w177:T16)  [unwired: 7 out]
                n86 = call-poly <instrlib>:"Signals (Set).vi"("error in"=w176, "PSU Act Stat"=w157, "Mercury Reference In"=w177) -> ("error out"=w159:errorcluster, "Response"=w169:T21)  [unwired: 1 in, 6 out]
                n87 = local write "Magnet Response"(w169) -> ()
                n88 = call-poly <instrlib>:"Open.vi"("error in (no error)"=w159, "Device Identifier"=T1 "GRPY" ("Device Identifier 2"), "Mercury Reference In"=w155) -> ("error out"=w165:errorcluster, "Mercury Reference Out"=w164:T16)  [unwired: 7 out]
                n89 = call-poly <instrlib>:"Signals (Set).vi"("error in"=w165, "PSU Act Stat"=w157, "Mercury Reference In"=w164) -> ("error out"=w158:errorcluster, "Response"=w167:T21)  [unwired: 1 in, 6 out]
                n90 = local write "Magnet Response"(w167) -> ()
                n91 = call-poly <instrlib>:"Open.vi"("error in (no error)"=w158, "Device Identifier"=T1 "GRPZ" ("Device Identifier 2"), "Mercury Reference In"=w155) -> ("error out"=w162:errorcluster, "Mercury Reference Out"=w163:T16)  [unwired: 7 out]
                n92 = call-poly <instrlib>:"Signals (Set).vi"("error in"=w162, "PSU Act Stat"=w157, "Mercury Reference In"=w163) -> ("error out"=w156:errorcluster, "Response"=w160:T21)  [unwired: 1 in, 6 out]
                n93 = local write "Magnet Response"(w160) -> ()
                n94 = call "FGV_PSP - VRM Actions.vi"("error in"=w156, "Function"=enum16{"write", "read"}."read") -> ("error out"=w173:errorcluster, "VRM actions"=w175:T8)  [unwired: 4 in]
                n95 = Bundle By Name(cluster=w175, "To Set"=w172) -> (w174:T8)
                n96 = local write "To Set"(w172) -> ()
                n97 = call "FGV_PSP - VRM Actions.vi"("error in"=w173, "Function"=enum16{"write", "read"}."write", "VRM actions"=w174) -> ("error out"=w171:errorcluster)  [unwired: 3 in, 1 out]
              }
            }
          }
          event "To Zero": Value Change {
            n98 = event-data() -> ()  [unwired: 1 in, 6 out]
            n99 = local read "To Zero"() -> (w178:bool)
            n100 = Unbundle By Name(w182) -> ("Mercury IPS Ref"=w179:T16)
            n101 = case shown="True" w178 {
              tunnel: [w184 w199] -> w181
              tunnel: w180 -> [w184 w197]
              tunnel: w179 -> [_ w187]
              frame False {
              }
              frame True {
                w200 = FALSE
                w188 = T20 "RTOZ" ("PSU Act Stat")
                n102 = call-poly <instrlib>:"Open.vi"("error in (no error)"=w197, "Device Identifier"=T1 "GRPX" ("Device Identifier 2"), "Mercury Reference In"=w187) -> ("error out"=w206:errorcluster, "Mercury Reference Out"=w207:T16)  [unwired: 7 out]
                n103 = call-poly <instrlib>:"Signals (Set).vi"("error in"=w206, "PSU Act Stat"=w188, "Mercury Reference In"=w207) -> ("error out"=w190:errorcluster, "Response"=w205:T21)  [unwired: 1 in, 6 out]
                n104 = local write "Magnet Response"(w205) -> ()
                n105 = call-poly <instrlib>:"Open.vi"("error in (no error)"=w190, "Device Identifier"=T1 "GRPY" ("Device Identifier 2")) -> ("error out"=w194:errorcluster)  [unwired: 1 in, 8 out]
                n106 = call-poly <instrlib>:"Signals (Set).vi"("error in"=w194, "PSU Act Stat"=w188, "Mercury Reference In"=w187) -> ("error out"=w189:errorcluster, "Response"=w195:T21)  [unwired: 1 in, 6 out]
                n107 = local write "Magnet Response"(w195) -> ()
                n108 = call-poly <instrlib>:"Open.vi"("error in (no error)"=w189, "Device Identifier"=T1 "GRPZ" ("Device Identifier 2")) -> ("error out"=w193:errorcluster)  [unwired: 1 in, 8 out]
                n109 = call-poly <instrlib>:"Signals (Set).vi"("error in"=w193, "PSU Act Stat"=w188, "Mercury Reference In"=w187) -> ("error out"=w186:errorcluster, "Response"=w192:T21)  [unwired: 1 in, 6 out]
                n110 = local write "Magnet Response"(w192) -> ()
                n111 = call "FGV_PSP - VRM Actions.vi"("error in"=w186, "Function"=enum16{"write", "read"}."read") -> ("error out"=w203:errorcluster, "VRM actions"=w201:T8)  [unwired: 4 in]
                n112 = Bundle By Name(cluster=w201, "To Zero"=w200) -> (w204:T8)
                n113 = local write "To Zero"(w200) -> ()
                n114 = call "FGV_PSP - VRM Actions.vi"("error in"=w203, "Function"=enum16{"write", "read"}."write", "VRM actions"=w204) -> ("error out"=w199:errorcluster)  [unwired: 3 in, 1 out]
              }
            }
          }
          event "Send to IPS": Value Change {
            n115 = event-data() -> ()  [unwired: 1 in, 6 out]
            n116 = local read "Send to IPS"() -> (w208:bool)
            n117 = Unbundle By Name(w212) -> ("Mercury IPS Ref"=w211:T16)
            n118 = case shown="True" w208 {
              tunnel: w211 -> [_ w233]
              tunnel: [w214 w216] -> w210
              tunnel: w209 -> [w214 w223]
              frame False {
              }
              frame True {
                w217 = FALSE ("Send to IPS")
                n119 = local read "X Setpoint (T)"() -> (w238:dbl)
                n120 = local read "Y Setpoint (T)"() -> (w237:dbl)
                n121 = local read "Z Setpoint (T)"() -> (w236:dbl)
                n122 = local read "X Field (T)"() -> (w246:dbl)
                n123 = local read "Y Field (T)"() -> (w245:dbl)
                n124 = local read "Z Field (T)"() -> (w244:dbl)
                n125 = local read "Sweep Rate (T/min)"() -> (w224:dbl)
                n126 = Bundle By Name(cluster=T9 {"Bx0 (T)"=0.0, "By0 (T)"=0.0, "Bz0 (T)"=0.0} ("B initial"), "Bx0 (T)"=w246, "By0 (T)"=w245, "Bz0 (T)"=w244) -> (w243:T9)
                n127 = Bundle By Name(cluster=T10 {"Bx (T)"=0.0, "By (T)"=0.0, "Bz (T)"=0.0} ("B target"), "Bx (T)"=w238, "By (T)"=w237, "Bz (T)"=w236) -> (w242:T10)
                n128 = call "CalculateSweepRate_xyz.vi"("Sweep rate (T/min)"=w224, "B target"=w242, "B initial"=w243) -> ("time (min)"=→"Time (min)":dbl, "Sweep Rates"=w226:T22)  [unwired: 6 in, 1 out]
                n129 = call-poly <instrlib>:"Open.vi"("error in (no error)"=w223, "Device Identifier"=T1 "GRPX" ("Device Identifier 2"), "Mercury Reference In"=w233) -> ("error out"=w263:errorcluster, "Mercury Reference Out"=w262:T16)  [unwired: 7 out]
                n130 = Unbundle By Name(w226) -> ("Rate_x (T/min)"=w241:dbl, "Rate_y (T/min)"=w240:dbl, "Rate_z (Tmin)"=w239:dbl)
                n131 = call-poly <instrlib>:"Signals (Set).vi"("error in"=w263, "Target Field"=w238, "Mercury Reference In"=w262) -> ("error out"=w261:errorcluster, "Response"=w232:T21, "Mercury Reference Out"=w260:T16)  [unwired: 2 in, 4 out]
                n132 = call-poly <instrlib>:"Signals (Set).vi"("error in"=w261, "Target Field Rate"=w241, "Mercury Reference In"=w260) -> ("error out"=w235:errorcluster, "Response"=w231:T21)  [unwired: 2 in, 5 out]
                n133 = call-poly <instrlib>:"Open.vi"("error in (no error)"=w235, "Device Identifier"=T1 "GRPY" ("Device Identifier 2"), "Mercury Reference In"=w233) -> ("error out"=w251:errorcluster, "Mercury Reference Out"=w257:T16)  [unwired: 7 out]
                n134 = call-poly <instrlib>:"Signals (Set).vi"("error in"=w251, "Target Field"=w237, "Mercury Reference In"=w257) -> ("error out"=w252:errorcluster, "Response"=w230:T21, "Mercury Reference Out"=w258:T16)  [unwired: 2 in, 4 out]
                n135 = call-poly <instrlib>:"Signals (Set).vi"("error in"=w252, "Target Field Rate"=w240, "Mercury Reference In"=w258) -> ("error out"=w234:errorcluster, "Response"=w229:T21)  [unwired: 2 in, 5 out]
                n136 = call-poly <instrlib>:"Open.vi"("error in (no error)"=w234, "Device Identifier"=T1 "GRPZ" ("Device Identifier 2"), "Mercury Reference In"=w233) -> ("error out"=w250:errorcluster, "Mercury Reference Out"=w255:T16)  [unwired: 7 out]
                n137 = call-poly <instrlib>:"Signals (Set).vi"("error in"=w250, "Target Field"=w236, "Mercury Reference In"=w255) -> ("error out"=w249:errorcluster, "Response"=w228:T21, "Mercury Reference Out"=w254:T16)  [unwired: 2 in, 4 out]
                n138 = call-poly <instrlib>:"Signals (Set).vi"("error in"=w249, "Target Field Rate"=w239, "Mercury Reference In"=w254) -> ("error out"=w218:errorcluster, "Response"=w227:T21)  [unwired: 2 in, 5 out]
                n139 = local write "Magnet Response"(w232) -> ()
                n140 = local write "Magnet Response"(w231) -> ()
                n141 = local write "Magnet Response"(w230) -> ()
                n142 = local write "Magnet Response"(w229) -> ()
                n143 = local write "Magnet Response"(w228) -> ()
                n144 = local write "Magnet Response"(w227) -> ()
                n145 = call "FGV_PSP - VRM Actions.vi"("error in"=w218, "Function"=enum16{"write", "read"}."read") -> ("error out"=w220:errorcluster, "VRM actions"=w219:T8)  [unwired: 4 in]
                n146 = local write "Send to IPS"(w217) -> ()
                n147 = Bundle By Name(cluster=w219, "Send to IPS"=w217) -> (w222:T8)
                n148 = call "FGV_PSP - VRM Actions.vi"("error in"=w220, "Function"=enum16{"write", "read"}."write", "VRM actions"=w222) -> ("error out"=w216:errorcluster)  [unwired: 3 in, 1 out]
              }
            }
          }
          event "OK": Value Change {
            # "Exit Button Value Change (pressed) Event\n(this executes Macro: Exit to terminate the VI)"
            n149 = event-data() -> ()  [unwired: 1 in, 1 out]
            n150 = call <vilib>:"Add State(s) to Queue__JKI_lib_State_Machine.vi"("State(s) in Front (\"\")"="Macro: Exit", "State(s) in (\"\")"=w268) -> ("States Out"=w267:string)  [unwired: 13 in]
          }
          event Panel Close? {
            # "Discard the event because we'll close the front panel ourselves in Macro: Exit"
            # "Close Panel button (pressed) Event\n(this executes Macro: Exit to terminate the VI)"
            n151 = event-data() -> ()  [unwired: 1 in, 1 out]
            n152 = call <vilib>:"Add State(s) to Queue__JKI_lib_State_Machine.vi"("State(s) in Front (\"\")"="Macro: Exit", "State(s) in (\"\")"=w274) -> ("States Out"=w273:string)  [unwired: 13 in]
            n153 = event-data("Discard?"=TRUE) -> ()  [unwired: 1 in, 1 out]
          }
        }
      }
      frame "---------- Core ----------" {
        # "Do not put any code in this frame.\n(it is a separator no-op)"
        n154 = call <vilib>:"Add State(s) to Queue__JKI_lib_State_Machine.vi"("State(s) in (\"\")"=w278) -> ("States Out"=w277:string)  [unwired: 14 in]
      }
      frame Default {
        w288 = 42 items=["No error", "Argument error", "Memory is full", "Out of zone", "End of file", "File already open", "Generic file I/O error", "File not found", "File permission error", "Disk is full", "Duplicate path", "Too many files open", "System feature not enabled", "Resource file not found", "Cannot add resource", "Resource not found", "Image not found", "Image memory error", "Pen does not exist", "Config type invalid", "Config token not found", "Config parse error", "Config memory error", "Bad external code format", "Bad external code offset", "External code not present", "Null window", "Destroy window error", "Null menu", "Print aborted", "Bad print record", "Print driver error", "Windows error during printing", "Memory error during printing", "Print dialog error", "Generic print error", "Invalid device refnum", "Device not found", "Device parameter error", "Device unit error", "Cannot open device", "Device call aborted", "Generic error", "Cancelled by user", "Object ID too low", "Object ID too high", "Object not in heap", "Unknown heap", "Unknown object (invalid DefProc)", "Unknown object (DefProc not in table)", "Message out of range", "Invalid (null) method", "Unknown message", "Manager call not supported", "Bad address", "Network operation in progress", "Network operation timed out", "Connection is busy", "Network attribute not supported", "Network error", "Address in use", "System out of memory", "Connection aborted", "Connection refused", "Not connected", "Already connected", "Connection closed", "Initialization error (interapplication manager)", "Bad occurrence", "Wait on unbound occurrence handler", "Occurrence queue overflow", "Datalog type conflict", "Unused", "Unrecognized type (interapplication manager)", "Memory corrupt", "Failed to make temporary DLL", "Old CIN version", "Drag socket not found", "Failed to load drop-object", "Failed to register OLE object", "Failed to release OLE object", "Format specifier type mismatch", "Unknown format specifier", "Too few format specifiers", "Too many format specifiers", "Scan failed", "Newer CIN version", "Error converting to variant", "Runtime menu error", "Password tampered", "Variant attribute not found", "Incompatible variant data type", "Event data is not available", "Event Store is not present", "Occurrence is not found", "Event Queue is not created", "Event info is not available", "Refnum passed is NULL", "Error retrieving Class GUID", "Error retrieving CoClass GUID", "Error retrieving TypeLib GUID.", "Bad built application magic bytes.", "Specific driver is different from the specific driver associated with the Logical Name.", "There is no session opened to the class driver.", "Max Error", "MAX - Error with config objects", "MAX - Error loading configuration", "MAX - Group not supported"]
        # "Current State"
        # "Do not delete, rename, or modify this frame.\n(this is used to capture unhandled states and typos)"
        # "Handle mistyped state name (developer tool)"
        n155 = Format Into String(format string="Software Exception: Unhandled State \"%s\"." ("message"), error in=w284, w279) -> (resulting string=w287:string, error out=w286:errorcluster)  [unwired: 1 in]
        n156 = call <vilib>:"Error Cluster From Error Code.vi"("show call chain? (False)"=TRUE, "error in (no error)"=w286, "error message (\"\")"=w287, "error code (0)"=w288) -> ("error out"=w285:errorcluster)  [unwired: 5 in]
        n157 = call <vilib>:"Add State(s) to Queue__JKI_lib_State_Machine.vi"("State(s) in (\"\")"=w283) -> ("States Out"=w282:string)  [unwired: 14 in]
      }
      frame "Initialize Core Data" {
        # "Do not delete, rename, or modify this frame.\n(this is used to determine panel behavior on exit)"
        # "originally closed?"
        # "exe?"
        # "If panel starts closed or is an EXE, then close it when we exit"
        n158 = property class="VI"() -> ("Front Panel.Open"=w297:bool)  [unwired: 2 in, 2 out]
        n159 = property class="App"() -> ("App.Kind"=w296:T11)  [unwired: 2 in, 2 out]
        n160 = control-ref of="Current VI Reference"() -> (w290:refnum<vi>)
        n161 = Not(x=w297) -> (.not. x?=w294:bool)
        n162 = Equal?(x=w296, y=T11."Run Time System" ("Application:Kind")) -> (x = y?=w293:bool)
        n163 = Or(x=w294, y=w293) -> (x .or. y?=w291:bool)
        n164 = Bundle By Name(cluster=w292, "Core.Current VI Reference"=w290, "Core.Close Panel on Exit?"=w291) -> (w299:T18)
        n165 = call <vilib>:"Add State(s) to Queue__JKI_lib_State_Machine.vi"("State(s) in (\"\")"=w301) -> ("States Out"=w300:string)  [unwired: 14 in]
      }
      frame "Error Handler" {
        w312 = i32[] [-1950679035, -1950678943]  # Error Codes to Filter
        # "Unhandled Error -- Display it"
        # "Handle any errors here.\nYou can also output any states to clean-up after errors occur"
        # "Clear error"
        n166 = call-poly <userlib>:"Filter Error Codes__ogtk.vi"("Error In"=w313, "Error Codes to Filter"=w312) -> ("Error Out"=w314:errorcluster, "Filtered Error Details"=w311:T23)  [unwired: 7 in, 1 out]
        n167 = Unbundle(w311) -> ("code"=w309:i32, "source"=w310:string)
        n168 = Get Date/Time In Seconds() -> (seconds since 1Jan1904=w308:timestamp)
        n169 = Unbundle By Name(w304) -> ("Error Log"=w306:T7)
        n170 = Bundle By Name(cluster=T12 {"time"=timestamp(0 s since 1904-01-01), "code"=0, "source"=""} ("output cluster"), "time"=w308, "code"=w309, "source"=w310) -> (w305:T12)
        n171 = Build Array (concatenate)(w306, w305) -> (w302:T7)
        "Error List" <- w302
        n172 = Bundle By Name(cluster=w304, "Error Log"=w302) -> (w303:T18)
        n173 = call <vilib>:"General Error Handler.vi"("error in (no error)"=w314) -> ()  [unwired: 10 in, 5 out]
        n174 = call <vilib>:"Add State(s) to Queue__JKI_lib_State_Machine.vi"("State(s) in Front (\"\")"="/* Post Error States", "State(s) in (\"\")"=w318) -> ("States Out"=w317:string)  [unwired: 13 in]
      }
      frame "Exit" {
        # "Do not put any code in this frame.\n(No errors that occur here will be handled.)"
        n175 = call <vilib>:"Add State(s) to Queue__JKI_lib_State_Machine.vi"("State(s) in (\"\")"=w323) -> ("States Out"=w322:string)  [unwired: 14 in]
      }
      frame "---------- Data ----------" {
        # "Do not put any code in this frame.\n(It is a separator no-op. You can make a copy of this frame to create a new Data frame)"
        n176 = call <vilib>:"Add State(s) to Queue__JKI_lib_State_Machine.vi"("State(s) in (\"\")"=w327) -> ("States Out"=w326:string)  [unwired: 14 in]
      }
      frame "Data: Initialize" {
        w328 = T7 []  # Error Log
        w330 = TRUE  # sentinel
        w331 = T16 {"Comms"="", "Device ID"=[], "Comms Layer"=enum."Ethernet TCP/IP", "Command"="", "Query reference"=refnum}  # Mercury IPS Ref
        w332 = T24 {"Current VI Reference"=refnum, "Close Panel on Exit?"=FALSE}  # Core
        # "do not delete - used by framework"
        # "Expand Bundle to add new data elements to shift register data."
        # "Add new data here."
        # "Data names and types of shift register data are defined by this bundle."
        # "Initialize the shift-register data, here.\n(data names are defined by what you wire into the bundle function)"
        n177 = Bundle("Core"=w332, "Mercury IPS Ref"=w331, "sentinel"=w330, "Error Log"=w328) -> (w333:T18)  [unwired: 1 in]
        n178 = call <vilib>:"Add State(s) to Queue__JKI_lib_State_Machine.vi"("State(s) in (\"\")"=w335) -> ("States Out"=w334:string)  [unwired: 14 in]
      }
      frame "Data: Cleanup" {
        # "Cleanup any data and references, here.\n(this is called automatically, by the Macro: Exit)"
        n179 = Unbundle By Name(w336) -> ("Core.Current VI Reference"=w339:refnum<vi>)
        n180 = Close Reference(reference=w339, error in (no error)=w338) -> (error out=w337:errorcluster)
        n181 = call <vilib>:"Add State(s) to Queue__JKI_lib_State_Machine.vi"("State(s) in (\"\")"=w341) -> ("States Out"=w340:string)  [unwired: 14 in]
      }
      frame "---------- UI ----------" {
        # "Do not put any code in this frame.\n(It is a separator no-op. You can make a copy of this frame to create a new UI frame)"
        n182 = call <vilib>:"Add State(s) to Queue__JKI_lib_State_Machine.vi"("State(s) in (\"\")"=w345) -> ("States Out"=w344:string)  [unwired: 14 in]
      }
      frame "UI: Initialize" {
        w360 = 0.0 ("X Target (T)")
        w365 = FALSE
        w358 = "" ("Magnet Status 2")
        # "start in local mode"
        # "Initialize the User Interface, here.\n(this is called automatically, by the Macro: Init)"
        n183 = Current VI's Path() -> (path=w353:path)
        n184 = Strip Path(path=w353) -> (stripped path=w352:path, name=w350:string)
        n185 = Concatenate Strings(w350, ".startup" ("name or relative path")) -> (w349:string)
        n186 = Build Path(base path=w352, name or relative path=w349) -> (appended path=w347:path)
        n187 = call "Read From Measurement File"("error in (no error)"=w355, "File Name"=w347) -> ("error out"=w356:errorcluster, "Signals"=w357:dynamicdata)  [unwired: 2 in, 6 out]
        n188 = case shown="No Error" w356 {
          selector: w356 -> [_ w376]
          tunnel: w357 -> [w374 _]
          tunnel: [_ w375] -> w348
          frame No Error {
            # "read last used values\nfrom startup file"
            n189 = Split Signals(w374) -> (w370:dynamicdata, w371:dynamicdata, w372:dynamicdata, w373:dynamicdata)  [unwired: 4 out]
            n190 = local write "Y Setpoint (T)"(w371) -> ()
            n191 = local write "Z Setpoint (T)"(w372) -> ()
            n192 = local write "X Setpoint (T)"(w370) -> ()
            n193 = local write "Sweep Rate (T/min)"(w373) -> ()
          }
          frame Error {
            # "if the file doesn't exist\ndon't worry, just clear the error"
            n194 = call <vilib>:"Clear Errors.vi"("error in (no error)"=w376) -> ("error out"=w375:errorcluster)  [unwired: 5 in, 1 out]
          }
        }
        n195 = local write "OK"(FALSE ("OK")) -> ()
        n196 = Open Application Reference(8:w348) -> (0:w361:errorcluster, 3:w364:refnum<vi>)  [unwired: 3 in]
        n197 = property class="App"(reference=w364, error in=w361, "WebSrvr.Active"=TRUE ("Web Server:Server Active")) -> (error out=w362:errorcluster)  [unwired: 1 out]
        n198 = call <vilib>:"Add State(s) to Queue__JKI_lib_State_Machine.vi"("State(s) in (\"\")"=w369) -> ("States Out"=w368:string)  [unwired: 14 in]
        n199 = local write "Remote Mode"(w365) -> ()
        n200 = call "FGV_PSP - VRM Remote.vi"("error in"=w362, "Function"=enum16{"write", "read"}."write", "VRM Remote"=w365) -> ("error out"=w354:errorcluster)  [unwired: 3 in, 1 out]
        n201 = local write "Error List"(T7 [] ("Error List")) -> ()
        "Magnet Response" <- w358
        "Y Target (T)" <- w360
        "Y Rate (T/min)" <- w360
        "Y Field (T)" <- w360
        "Z Target (T)" <- w360
        "Z Rate (T/min)" <- w360
        "Z Field (T)" <- w360
        "Z Current (A)" <- w360
        "Z Voltage (V)" <- w360
        "Phi Field (deg)" <- w360
        "Phi Target (deg)" <- w360
        "Y Current (A)" <- w360
        "Y Voltage (V)" <- w360
        "Theta Field (deg)" <- w360
        "X Current (A)" <- w360
        "X Voltage (V)" <- w360
        "R Field (T)" <- w360
        "X Field (T)" <- w360
        "X Target (T)" <- w360
        "R Target (T)" <- w360
        "X Rate (T/min)" <- w360
        "Theta Target (deg)" <- w360
        "X Magnet Status" <- w358
        "Y Magnet Status" <- w358
        "Z Magnet Status" <- w358
      }
      frame "UI: Cursor Set" {
        # "Argument"
        # "Set and Unset Cursor Busy.\n(Usage: \"UI: Cursor Set >> Busy|Idle\")"
        n202 = case shown="\"Idle\", Default" w377 {
          tunnel: w379 -> [w384 w386]
          tunnel: [w383 w385] -> w378
          frame "Idle", Default {
            n203 = call <vilib>:"Unset Busy.vi"("error in (no error)"=w384) -> ("error out"=w383:errorcluster)  [unwired: 10 in]
          }
          frame "Busy" {
            n204 = call <vilib>:"Set Busy.vi"("error in (no error)"=w386) -> ("error out"=w385:errorcluster)  [unwired: 9 in, 1 out]
          }
        }
        n205 = call <vilib>:"Add State(s) to Queue__JKI_lib_State_Machine.vi"("State(s) in (\"\")"=w382) -> ("States Out"=w381:string)  [unwired: 14 in]
      }
      frame "UI: Front Panel State" {
        # "Argument"
        # "Set Front Panel Open or Closed\n(Usage: \"UI: Front Panel State >> Open|Close\")"
        n206 = Unbundle By Name(w389) -> ("Core.Current VI Reference"=w388:refnum<vi>)
        n207 = case shown="\"Open\", Default" w387 {
          tunnel: w391 -> [w397 w410]
          tunnel: [w399 w411] -> w390
          tunnel: w388 -> [w398 w408]
          frame "Open", Default {
            n208 = property class="VI"(reference=w398, error in=w397) -> (reference out=w395:refnum<vi>, error out=w396:errorcluster, "Front Panel.Open"=w394:bool)
            n209 = case shown="True" w394 {
              tunnel: [w402 w405] -> w399
              tunnel: w396 -> [w401 w405]
              tunnel: w395 -> [w400 _]
              frame False {
                n210 = invoke class="VI" method="FP.Open"(reference=w400, error in=w401, "Activate"=TRUE, "State"=T13."Standard") -> (error out=w402:errorcluster)  [unwired: 1 in, 4 out]
              }
              frame True {
              }
            }
          }
          frame "Close" {
            n211 = property class="VI"(reference=w408, error in=w410) -> (reference out=w407:refnum<vi>, error out=w409:errorcluster, "Front Panel.Open"=w406:bool)
            n212 = case shown="True" w406 {
              tunnel: [w412 w415] -> w411
              tunnel: w409 -> [w412 w414]
              tunnel: w407 -> [_ w413]
              frame False {
              }
              frame True {
                n213 = invoke class="VI" method="FP.Close"(reference=w413, error in=w414) -> (error out=w415:errorcluster)  [unwired: 1 in, 2 out]
              }
            }
          }
        }
        n214 = call <vilib>:"Add State(s) to Queue__JKI_lib_State_Machine.vi"("State(s) in (\"\")"=w393) -> ("States Out"=w392:string)  [unwired: 14 in]
      }
      frame "---------- Macro ----------" {
        # "Do not put any code in this frame.\n(It is a separator no-op. You can make a copy of this frame to create a new Macro frame)"
        n215 = call <vilib>:"Add State(s) to Queue__JKI_lib_State_Machine.vi"("State(s) in (\"\")"=w419) -> ("States Out"=w418:string)  [unwired: 14 in]
      }
      frame "Macro: Initialize" {
        w420 = "Data: Initialize\nInitialize Core Data\nUI: Initialize\nUI: Front Panel State >> Open\nMercury: Initialize"  # Data: Initialize Initialize Core Data UI: Initialize UI: Front Panel State >> Open Mercury: Initialize
        # "Initialization Macro\n(This is called once, when the VI starts)"
        n216 = call <vilib>:"Add State(s) to Queue__JKI_lib_State_Machine.vi"("State(s) in Front (\"\")"=w420, "State(s) in (\"\")"=w424) -> ("States Out"=w423:string)  [unwired: 13 in]
      }
      frame "Macro: Exit" {
        # "Exit Macro\n(This is called once, when the VI exits)"
        n217 = Unbundle By Name(w448) -> ("Core.Close Panel on Exit?"=w447:bool, "Mercury IPS Ref"=w440:T16)
        n218 = call <instrlib>:"Close.vi"("error in (no error)"=w441, "Mercury Reference"=w440) -> ("error out"=w439:errorcluster)  [unwired: 9 out]
        n219 = call <vilib>:"Simple Error Handler.vi"("error in (no error)"=w439) -> ("error out"=w431:errorcluster)  [unwired: 1 in, 7 out]
        n220 = Current VI's Path() -> (path=w430:path)
        n221 = Strip Path(path=w430) -> (stripped path=w429:path, name=w427:string)
        n222 = Concatenate Strings(w427, ".startup" ("name or relative path")) -> (w426:string)
        n223 = Build Path(base path=w429, name or relative path=w426) -> (appended path=w432:path)
        n224 = local read "X Setpoint (T)"() -> (w437:dbl)
        n225 = local read "Y Setpoint (T)"() -> (w436:dbl)
        n226 = local read "Z Setpoint (T)"() -> (w435:dbl)
        n227 = local read "Sweep Rate (T/min)"() -> (w434:dbl)
        n228 = local write "OK"(FALSE ("OK")) -> ()
        n229 = Select(t="UI: Front Panel State >> Close", s=w447, f="") -> (s? t:f=w444:string)
        n230 = call <vilib>:"Add State(s) to Queue__JKI_lib_State_Machine.vi"("State(s) in (\"\")"=w444, "State(s) at Back (\"\")"="Data: Cleanup\nExit") -> ("States Out"=w442:string)  [unwired: 13 in]
        n231 = Merge Signals(w437, w436, w435, w434) -> (w438:dynamicdata)
        n232 = call "Write To Measurement File"("Signals"=w438, "error in (no error)"=w431, "File Name"=w432) -> ("error out"=w433:errorcluster)  [unwired: 4 in, 12 out]
        n233 = call <vilib>:"Add State(s) to Queue__JKI_lib_State_Machine.vi"("State(s) in Front (\"\")"=w442, "State(s) in (\"\")"=w450) -> ("States Out"=w449:string)  [unwired: 13 in]
      }
      frame "---------- New Category ----------" {
        n234 = call <vilib>:"Add State(s) to Queue__JKI_lib_State_Machine.vi"("State(s) in (\"\")"=w454) -> ("States Out"=w453:string)  [unwired: 14 in]
      }
      frame "Mercury: Initialize" {
        n235 = call-poly <instrlib>:"Open.vi"("Clear Previous Connections (False)"=TRUE ("Clear Previous Connections (True)"), "ID Query (True)"=TRUE, "IP Address"="IPS IP Address", "error in (no error)"=w455, "Comms Layer"=Comms_Transport_Layer."Ethernet TCP/IP") -> ("error out"=w458:errorcluster, "# of Instruments"=→"# of Instruments":i32, "Serial Number(s)"=→"Serial Number(s)":string[], "Mercury Reference Out"=w457:T16, "S/W Version(s)"=→"S/W Version(s)":string[])  [unwired: 2 in]
        n236 = Bundle By Name(cluster=w467, "Mercury IPS Ref"=w457) -> (w466:T18)
        n237 = call <vilib>:"Add State(s) to Queue__JKI_lib_State_Machine.vi"("State(s) in (\"\")"=w469, "State(s) at Back (\"\")"="Mercury: Query IPS: System\nMercury: Query IPS: Magnet" ("State(s) at Back (\"\")")) -> ("States Out"=w468:string)  [unwired: 13 in]
      }
      frame "Mercury: Query IPS: System" {
        n238 = Unbundle By Name(w511) -> ("Mercury IPS Ref"=w470:T16)
        n239 = call-poly <instrlib>:"Configuration (Read).vi"("error in"=w477, "Mercury Reference In"=w470) -> ("error out"=w497:errorcluster, "Devices"=→"IPS Devices":string[], "Mercury Reference Out"=w496:T16)  [unwired: 1 in, 6 out]
        n240 = call-poly <instrlib>:"Configuration (Read).vi"("error in"=w497, "Mercury Reference In"=w496) -> ("error out"=w501:errorcluster, "Automatic Dimming"=→"Automatic Dimming":string, "Mercury Reference Out"=w500:T16)  [unwired: 1 in, 6 out]
        n241 = call-poly <instrlib>:"Configuration (Read).vi"("error in"=w501, "Mercury Reference In"=w500) -> ("error out"=w498:errorcluster, "Dimming Time"=→"Dimming Time":string, "Mercury Reference Out"=w499:T16)  [unwired: 1 in, 6 out]
        n242 = call-poly <instrlib>:"Configuration (Read).vi"("error in"=w498, "Mercury Reference In"=w499) -> ("error out"=w495:errorcluster, "Display Brightness"=→"Display Brightness":string, "Mercury Reference Out"=w494:T16)  [unwired: 1 in, 6 out]
        n243 = call-poly <instrlib>:"Configuration (Read).vi"("error in"=w495, "Mercury Reference In"=w494) -> ("error out"=w504:errorcluster, "Date"=→"Date":string, "Mercury Reference Out"=w505:T16)  [unwired: 1 in, 6 out]
        n244 = call-poly <instrlib>:"Configuration (Read).vi"("error in"=w504, "Mercury Reference In"=w505) -> ("error out"=w502:errorcluster, "Time"=→"Time":string, "Mercury Reference Out"=w503:T16)  [unwired: 1 in, 6 out]
        n245 = call-poly <instrlib>:"Configuration (Read).vi"("error in"=w502, "Mercury Reference In"=w503) -> ("error out"=w476:errorcluster, "time stamp"=→"time stamp":timestamp, "Mercury Reference Out"=w473:T16)  [unwired: 1 in, 6 out]
        n246 = call-poly <instrlib>:"Configuration (Read).vi"("error in"=w476, "Mercury Reference In"=w473) -> ("error out"=w478:errorcluster, "Hardware Version"=→"Hardware Version":string, "Mercury Reference Out"=w479:T16)  [unwired: 1 in, 6 out]
        n247 = call-poly <instrlib>:"Configuration (Read).vi"("error in"=w478, "Mercury Reference In"=w479) -> ("error out"=w480:errorcluster, "Firmware Version"=→"Firmware Version":string, "Mercury Reference Out"=w481:T16)  [unwired: 1 in, 6 out]
        n248 = call-poly <instrlib>:"Configuration (Read).vi"("error in"=w480, "Mercury Reference In"=w481) -> ("error out"=w486:errorcluster, "Serial Number"=→"Serial Number":string, "Mercury Reference Out"=w487:T16)  [unwired: 1 in, 6 out]
        n249 = call-poly <instrlib>:"Configuration (Read).vi"("error in"=w486, "Mercury Reference In"=w487) -> ("error out"=w482:errorcluster, "Free Space"=→"Free Space 2":i32, "Mercury Reference Out"=w483:T16)  [unwired: 1 in, 6 out]
        n250 = call-poly <instrlib>:"Configuration (Read).vi"("error in"=w482, "Mercury Reference In"=w483) -> ("error out"=w485:errorcluster, "Mode"=→"String 2":T25, "Mercury Reference Out"=w484:T16)  [unwired: 1 in, 6 out]
        n251 = Get Date/Time In Seconds() -> (seconds since 1Jan1904=w493:timestamp)
        n252 = call-poly <instrlib>:"Configuration (Set).vi"("error in"=w485, "time stamp"=w493, "Mercury Reference In"=w484) -> ("error out"=w475:errorcluster, "Response"=→"Set Date Response":T21)  [unwired: 1 in, 6 out]
        n253 = call <vilib>:"Add State(s) to Queue__JKI_lib_State_Machine.vi"("State(s) in (\"\")"=w513) -> ("States Out"=w512:string)  [unwired: 14 in]
      }
      frame "Mercury: Query IPS: Magnet" {
        n254 = Unbundle By Name(w552) -> ("Mercury IPS Ref"=w518:T16)
        n255 = call-poly <instrlib>:"Open.vi"("error in (no error)"=w515, "Device Identifier"=T1 "GRPX", "Mercury Reference In"=w518) -> ("error out"=w537:errorcluster, "Mercury Reference Out"=w536:T16)  [unwired: 7 out]
        n256 = call-poly <instrlib>:"Configuration (Read).vi"("error in"=w537, "Mercury Reference In"=w536) -> ("error out"=w540:errorcluster, "Magnet Device Details"=→"Magnet Device Details":T3, "Mercury Reference Out"=w539:T16)  [unwired: 1 in, 6 out]
        n257 = call-poly <instrlib>:"Configuration (Read).vi"("error in"=w540, "Mercury Reference In"=w539) -> ("error out"=w543:errorcluster, "Serial Number"=→"Mag S/N":string, "Mercury Reference Out"=w542:T16)  [unwired: 1 in, 6 out]
        n258 = call-poly <instrlib>:"Configuration (Read).vi"("error in"=w543, "Mercury Reference In"=w542) -> ("error out"=w546:errorcluster, "Bipolar Output"=→"Bipolar Output":string, "Mercury Reference Out"=w545:T16)  [unwired: 1 in, 6 out]
        n259 = call-poly <instrlib>:"Configuration (Read).vi"("error in"=w546, "Mercury Reference In"=w545) -> ("error out"=w549:errorcluster, "Out Config"=→"Out Config":T26, "Mercury Reference Out"=w548:T16)  [unwired: 1 in, 6 out]
        n260 = call-poly <instrlib>:"Configuration (Read).vi"("error in"=w549, "Mercury Reference In"=w548) -> ("error out"=w520:errorcluster, "Unit"=→"Unit 8":T6, "Current Limit"=→"Current Limit":dbl, "Mercury Reference Out"=w517:T16)  [unwired: 1 in, 5 out]
        n261 = call-poly <instrlib>:"Configuration (Read).vi"("error in"=w520, "Mercury Reference In"=w517) -> ("error out"=w523:errorcluster, "Unit"=→"Unit 9":T6, "AtoB"=→"AtoB":dbl, "Mercury Reference Out"=w522:T16)  [unwired: 1 in, 5 out]
        n262 = call-poly <instrlib>:"Configuration (Read).vi"("error in"=w523, "Mercury Reference In"=w522) -> ("error out"=w526:errorcluster, "Switch Present"=→"Switch Present":string, "Mercury Reference Out"=w525:T16)  [unwired: 1 in, 6 out]
        n263 = call-poly <instrlib>:"Configuration (Read).vi"("error in"=w526, "Mercury Reference In"=w525) -> ("error out"=w531:errorcluster, "Unit"=→"Unit 10":T6, "SW VLIM"=→"SW VLIM":dbl, "Mercury Reference Out"=w530:T16)  [unwired: 1 in, 5 out]
        n264 = call-poly <instrlib>:"Signals (Read).vi"("error in"=w531, "Mercury Reference In"=w530) -> ("error out"=w533:errorcluster, "Unit"=→"Unit 11":T6, "Current Rate"=→"Current Rate":dbl, "Mercury Reference Out"=w532:T16)  [unwired: 1 in, 5 out]
        n265 = call-poly <instrlib>:"Signals (Read).vi"("error in"=w533, "Mercury Reference In"=w532) -> ("error out"=w519:errorcluster, "PSU Act Stat"=→"PSU Act Stat":T20)  [unwired: 1 in, 7 out]
        n266 = call <vilib>:"Add State(s) to Queue__JKI_lib_State_Machine.vi"("State(s) in (\"\")"=w553) -> ("States Out"=w554:string)  [unwired: 14 in]
      }
      frame "Mercury: IPS: Idle - 1" {
        w570 = enum16{"write", "read"}."write" ("Function")
        n267 = Unbundle By Name(w633) -> ("Mercury IPS Ref"=w555:T16)
        n268 = call-poly <instrlib>:"Configuration (Read).vi"("error in"=w632, "Mercury Reference In"=w555) -> ("error out"=w629:errorcluster, "Time"=w631:string, "Mercury Reference Out"=w630:T16)  [unwired: 1 in, 6 out]
        n269 = local write "Time"(w631) -> ()
        n270 = call-poly <instrlib>:"Open.vi"("error in (no error)"=w629, "Device Identifier"=T1 "GRPX" ("Device Identifier 2"), "Mercury Reference In"=w630) -> ("error out"=w628:errorcluster, "Mercury Reference Out"=w622:T16)  [unwired: 1 in, 6 out]
        n271 = call-poly <instrlib>:"Signals (Read).vi"("error in"=w628, "Mercury Reference In"=w622) -> ("error out"=w627:errorcluster, "Target Field"=w581:dbl, "Mercury Reference Out"=w621:T16)  [unwired: 1 in, 6 out]
        n272 = call-poly <instrlib>:"Signals (Read).vi"("error in"=w627, "Mercury Reference In"=w621) -> ("error out"=w626:errorcluster, "Field"=w560:dbl, "Mercury Reference Out"=w620:T16)  [unwired: 1 in, 6 out]
        n273 = call-poly <instrlib>:"Signals (Read).vi"("error in"=w626, "Mercury Reference In"=w620) -> ("error out"=w625:errorcluster, "Target Field Rate"=w578:dbl, "Mercury Reference Out"=w619:T16)  [unwired: 1 in, 6 out]
        n274 = call-poly <instrlib>:"Signals (Read).vi"("error in"=w625, "Mercury Reference In"=w619) -> ("error out"=w624:errorcluster, "Current"=w573:dbl, "Mercury Reference Out"=w618:T16)  [unwired: 1 in, 6 out]
        n275 = call-poly <instrlib>:"Signals (Read).vi"("error in"=w624, "Mercury Reference In"=w618) -> ("error out"=w623:errorcluster, "Voltage"=w582:dbl, "Mercury Reference Out"=w617:T16)  [unwired: 1 in, 6 out]
        n276 = call-poly <instrlib>:"Signals (Read).vi"("error in"=w623, "Mercury Reference In"=w617) -> ("error out"=w572:errorcluster, "PSU Act Stat"=w564:T20)  [unwired: 1 in, 7 out]
        n277 = call-poly <instrlib>:"Open.vi"("error in (no error)"=w572, "Device Identifier"=T1 "GRPY" ("Device Identifier 2"), "Mercury Reference In"=w555) -> ("error out"=w615:errorcluster, "Mercury Reference Out"=w589:T16)  [unwired: 7 out]
        n278 = call-poly <instrlib>:"Signals (Read).vi"("error in"=w615, "Mercury Reference In"=w589) -> ("error out"=w614:errorcluster, "Target Field"=w580:dbl, "Mercury Reference Out"=w590:T16)  [unwired: 1 in, 6 out]
        n279 = call-poly <instrlib>:"Signals (Read).vi"("error in"=w614, "Mercury Reference In"=w590) -> ("error out"=w613:errorcluster, "Field"=w561:dbl, "Mercury Reference Out"=w591:T16)  [unwired: 1 in, 6 out]
        n280 = call-poly <instrlib>:"Signals (Read).vi"("error in"=w613, "Mercury Reference In"=w591) -> ("error out"=w612:errorcluster, "Target Field Rate"=w577:dbl, "Mercury Reference Out"=w592:T16)  [unwired: 1 in, 6 out]
        n281 = call-poly <instrlib>:"Signals (Read).vi"("error in"=w612, "Mercury Reference In"=w592) -> ("error out"=w611:errorcluster, "Current"=w574:dbl, "Mercury Reference Out"=w593:T16)  [unwired: 1 in, 6 out]
        n282 = call-poly <instrlib>:"Signals (Read).vi"("error in"=w611, "Mercury Reference In"=w593) -> ("error out"=w610:errorcluster, "Voltage"=w584:dbl, "Mercury Reference Out"=w594:T16)  [unwired: 1 in, 6 out]
        n283 = call-poly <instrlib>:"Signals (Read).vi"("error in"=w610, "Mercury Reference In"=w594) -> ("error out"=w588:errorcluster, "PSU Act Stat"=w563:T20)  [unwired: 1 in, 7 out]
        n284 = call-poly <instrlib>:"Open.vi"("error in (no error)"=w588, "Device Identifier"=T1 "GRPZ" ("Device Identifier 2"), "Mercury Reference In"=w555) -> ("error out"=w609:errorcluster, "Mercury Reference Out"=w600:T16)  [unwired: 7 out]
        n285 = call-poly <instrlib>:"Signals (Read).vi"("error in"=w609, "Mercury Reference In"=w600) -> ("error out"=w608:errorcluster, "Target Field"=w579:dbl, "Mercury Reference Out"=w599:T16)  [unwired: 1 in, 6 out]
        n286 = call-poly <instrlib>:"Signals (Read).vi"("error in"=w608, "Mercury Reference In"=w599) -> ("error out"=w607:errorcluster, "Field"=w559:dbl, "Mercury Reference Out"=w598:T16)  [unwired: 1 in, 6 out]
        n287 = call-poly <instrlib>:"Signals (Read).vi"("error in"=w607, "Mercury Reference In"=w598) -> ("error out"=w606:errorcluster, "Target Field Rate"=w576:dbl, "Mercury Reference Out"=w597:T16)  [unwired: 1 in, 6 out]
        n288 = call-poly <instrlib>:"Signals (Read).vi"("error in"=w606, "Mercury Reference In"=w597) -> ("error out"=w605:errorcluster, "Current"=w575:dbl, "Mercury Reference Out"=w596:T16)  [unwired: 1 in, 6 out]
        n289 = call-poly <instrlib>:"Signals (Read).vi"("error in"=w605, "Mercury Reference In"=w596) -> ("error out"=w604:errorcluster, "Voltage"=w583:dbl, "Mercury Reference Out"=w595:T16)  [unwired: 1 in, 6 out]
        n290 = call-poly <instrlib>:"Signals (Read).vi"("error in"=w604, "Mercury Reference In"=w595) -> ("error out"=w603:errorcluster, "PSU Act Stat"=w562:T20)  [unwired: 1 in, 7 out]
        n291 = local write "X Rate (T/min)"(w578) -> ()
        n292 = local write "Y Rate (T/min)"(w577) -> ()
        n293 = local write "Z Rate (T/min)"(w576) -> ()
        n294 = local write "X Current (A)"(w573) -> ()
        n295 = local write "Y Current (A)"(w574) -> ()
        n296 = local write "Z Current (A)"(w575) -> ()
        n297 = local write "X Voltage (V)"(w582) -> ()
        n298 = local write "Y Voltage (V)"(w584) -> ()
        n299 = local write "Z Voltage (V)"(w583) -> ()
        n300 = local write "X Target (T)"(w581) -> ()
        n301 = local write "Y Target (T)"(w580) -> ()
        n302 = local write "Z Target (T)"(w579) -> ()
        n303 = local write "X Field (T)"(w560) -> ()
        n304 = local write "Y Field (T)"(w561) -> ()
        n305 = local write "Z Field (T)"(w559) -> ()
        n306 = call "VRM_parse_status.vi"("PSU Act Stat"=w564) -> ("String"=w566:string)  [unwired: 10 in]
        n307 = call "VRM_parse_status.vi"("PSU Act Stat"=w563) -> ("String"=w567:string)  [unwired: 10 in]
        n308 = call "FGV_PSP - VRM Status.vi"("error in"=w603, "Function"=enum16{"write", "read"}."read") -> ("error out"=w586:errorcluster, "VRM status"=w585:T27)  [unwired: 4 in]
        n309 = local write "X Magnet Status"(w566) -> ()
        n310 = call "VRM_parse_status.vi"("PSU Act Stat"=w562) -> ("String"=w568:string)  [unwired: 10 in]
        n311 = Bundle By Name(cluster=w585, "X Target (T)"=w581, "Y Target (T)"=w580, "Z Target (T)"=w579, "X Field (T)"=w560, "Y Field (T)"=w561, "Z Field (T)"=w559, "X Rate (T/min)"=w578, "Y Rate (T/min)"=w577, "Z Rate (T/min)"=w576, "X Current (A)"=w573, "Y Current (A)"=w574, "Z Current (A)"=w575, "X Voltage (V)"=w582, "Y Voltage (V)"=w584, "Z Voltage (V)"=w583) -> (w569:T27)
        n312 = local write "Y Magnet Status"(w567) -> ()
        n313 = local write "Z Magnet Status"(w568) -> ()
        n314 = call "FGV_PSP - VRM Status.vi"("error in"=w586, "Function"=w570, "VRM status"=w569) -> ("error out"=w571:errorcluster)  [unwired: 3 in, 1 out]
        n315 = Build Array(w560, w561, w559) -> ()  [unwired: 1 out]
        n316 = Bundle By Name(cluster=T15 {"x action"="", "y action"="", "z action"=""} ("VRM Actions"), "x action"=w564, "y action"=w563, "z action"=w562) -> (w558:T15)
        n317 = call <vilib>:"Add State(s) to Queue__JKI_lib_State_Machine.vi"("State(s) in (\"\")"=w634) -> ("States Out"=w635:string)  [unwired: 14 in]
        n318 = call "FGV_PSP - VRM Action Status.vi"("error in"=w571, "Function"=w570, "VRM Actions"=w558) -> ("error out"=w557:errorcluster)  [unwired: 3 in, 1 out]
        n319 = call "VRM_to_DSC.vi"("error in (no error)"=w557, "VRM Actions"=w558, "VRM status"=w569) -> ("error out"=w556:errorcluster)  [unwired: 4 in]
      }
      frame "Mercury: IPS: Idle - 2" {
        w654 = u16 0 items=["Cartesian to spherical", "spherical to Cartesian", "Cartesian to cylindrical", "cylindrical to Cartesian", "spherical to cylindrical", "cylindrical to spherical"] ("conversion type")
        w652 = u16 0 items=["Cartesian to spherical", "spherical to Cartesian", "Cartesian to cylindrical", "cylindrical to Cartesian", "spherical to cylindrical", "cylindrical to spherical"] ("conversion type")
        n320 = Unbundle By Name(w658) -> ()  [unwired: 1 out]
        n321 = local read "X Target (T)"() -> (w651:dbl)
        n322 = local read "Y Target (T)"() -> (w650:dbl)
        n323 = local read "Z Target (T)"() -> (w649:dbl)
        n324 = local read "X Field (T)"() -> (w648:dbl)
        n325 = local read "Y Field (T)"() -> (w647:dbl)
        n326 = local read "Z Field (T)"() -> (w646:dbl)
        n327 = call-poly <vilib>:"3D Coordinate Conversion.vi"("conversion type"=w652, "axis 3"=w649, "axis 2"=w650, "axis 1"=w651) -> ("axis 3 out"=w656:dbl, "axis 2 out"=w657:dbl, "axis 1 out"=w642:dbl)  [unwired: 4 in, 1 out]
        n328 = call-poly <vilib>:"3D Coordinate Conversion.vi"("conversion type"=w654, "axis 3"=w646, "axis 2"=w647, "axis 1"=w648) -> ("axis 3 out"=w655:dbl, "axis 2 out"=w653:dbl, "axis 1 out"=w643:dbl)  [unwired: 4 in, 1 out]
        n329 = expression code="x*180/pi"(w657) -> (w636:dbl)
        n330 = expression code="x*180/pi"(w656) -> (w637:dbl)
        n331 = expression code="x*180/pi"(w653) -> (w639:dbl)
        n332 = expression code="x*180/pi"(w655) -> (w638:dbl)
        n333 = local write "Phi Target (deg)"(w637) -> ()
        n334 = local write "R Target (T)"(w642) -> ()
        n335 = local write "Theta Target (deg)"(w636) -> ()
        n336 = local write "R Field (T)"(w643) -> ()
        n337 = local write "Theta Field (deg)"(w639) -> ()
        n338 = local write "Phi Field (deg)"(w638) -> ()
        n339 = call "MakeXYZAxes.vi"("Field Magnitude"=w643, "Field Phi"=w638, "Field Theta"=w639, "Target Magnitude"=w642, "Target Phi"=w637, "Target Theta"=w636, "error in (no error)"=w645) -> ("error out"=w644:errorcluster, "Field Graph"=→"3D Graph":refnum<vi>, "Legend"=→"Legend":refnum<vi>)  [unwired: 10 in]
        n340 = call <vilib>:"Add State(s) to Queue__JKI_lib_State_Machine.vi"("State(s) in (\"\")"=w659) -> ("States Out"=w660:string)  [unwired: 14 in]
      }
      frame "Mercury: IPS: Idle - 3" {
        n341 = Unbundle By Name(w667) -> ("Mercury IPS Ref"=w665:T16)
        n342 = call-poly <instrlib>:"Open.vi"("Device Identifier"="Device Identifier 2", "Mercury Reference In"=w665) -> ("error out"=w662:errorcluster, "Mercury Reference Out"=w663:T16)  [unwired: 2 in, 6 out]
        n343 = call-poly <instrlib>:"Configuration (Read).vi"("error in"=w662, "Mercury Reference In"=w663) -> ("Firmware Version"=→"Firmware Version 2":string)  [unwired: 6 in, 3 out]
        n344 = call <vilib>:"Add State(s) to Queue__JKI_lib_State_Machine.vi"("State(s) in (\"\")"=w668) -> ("States Out"=w669:string)  [unwired: 14 in]
      }
    }
    "error out" <- w3
  }
  n345 = disable-structure shown="Disabled" {
    frame Disabled {
      n346 = local read "Remote Mode"() -> (w672:bool)
      n347 = case shown="True" w672 {
        tunnel: [_ w676] -> _
        tunnel: [_ w675] -> _
        frame False {
        }
        frame True {
          n348 = call "FGV_PSP - VRM Targets.vi"("Function"=enum16{"write", "read"}."read") -> ("VRM Targets 2"=w673:T19)  [unwired: 5 in, 1 out]
          n349 = Unbundle(w673) -> ("X Setpoint (T)"=w676:dbl, "Y Setpoint (T)"=w675:dbl)  [unwired: 2 out]
        }
      }
      n350 = local read "Send to IPS"() -> ()  [unwired: 1 out]
      n351 = call "FGV_PSP - VRM Targets.vi"("Function"=enum16{"write", "read"}."write") -> ()  [unwired: 5 in, 2 out]
      n352 = local write "Send to IPS"(FALSE) -> ()
    }
    frame Enabled {
    }
  }
  n353 = while {
    stop <- w679 stop-if-true
    n354 = local read "Remote Mode"() -> (w678:bool)
    n355 = case shown="False" w678 {
      frame False {
        n356 = local read "Tab Control 2"() -> (w680:enum32{"Cartesian", "Spherical"})
        n357 = case shown="\"Spherical\"" w680 {
          frame "Cartesian", Default {
            w681 = u16 0 items=["Cartesian to Spherical", "Spherical to Cartesian", "Cartesian to Cylindrical", "Cylindrical to Cartesian", "Spherical to Cylindrical", "Cylindrical to Spherical"] ("conversion type")
            n358 = local read "X Setpoint (T)"() -> (w686:dbl)
            n359 = local read "Y Setpoint (T)"() -> (w685:dbl)
            n360 = local read "Z Setpoint (T)"() -> (w684:dbl)
            n361 = call-poly <vilib>:"3D Coordinate Conversion.vi"("conversion type"=w681, "axis 3"=w684, "axis 2"=w685, "axis 1"=w686) -> ("axis 3 out"=w682:dbl, "axis 2 out"=w683:dbl, "axis 1 out"=w687:dbl)  [unwired: 4 in, 1 out]
            n362 = expression code="x*180/pi"(w682) -> (w689:dbl)
            n363 = expression code="x*180/pi"(w683) -> (w688:dbl)
            n364 = local write "R Setpoint (T)"(w687) -> ()
            n365 = local write "Theta Setpoint (deg)"(w688) -> ()
            n366 = local write "Phi Setpoint (deg)"(w689) -> ()
          }
          frame "Spherical" {
            w695 = u16 1 items=["Cartesian to Spherical", "Spherical to Cartesian", "Cartesian to Cylindrical", "Cylindrical to Cartesian", "Spherical to Cylindrical", "Cylindrical to Spherical"] ("conversion type")
            n367 = local read "Phi Setpoint (deg)"() -> (w698:dbl)
            n368 = local read "R Setpoint (T)"() -> (w694:dbl)
            n369 = local read "Theta Setpoint (deg)"() -> (w697:dbl)
            n370 = expression code="x*pi/180"(w698) -> (w693:dbl)
            n371 = expression code="x*pi/180"(w697) -> (w696:dbl)
            n372 = call-poly <vilib>:"3D Coordinate Conversion.vi"("conversion type"=w695, "axis 3"=w693, "axis 2"=w696, "axis 1"=w694) -> ("axis 3 out"=w692:dbl, "axis 2 out"=w691:dbl, "axis 1 out"=w690:dbl)  [unwired: 4 in, 1 out]
            n373 = local write "X Setpoint (T)"(w690) -> ()
            n374 = local write "Y Setpoint (T)"(w691) -> ()
            n375 = local write "Z Setpoint (T)"(w692) -> ()
          }
        }
      }
      frame True {
        w699 = u16 0 items=["Cartesian to Spherical", "Spherical to Cartesian", "Cartesian to Cylindrical", "Cylindrical to Cartesian", "Spherical to Cylindrical", "Cylindrical to Spherical"] ("conversion type")
        n376 = local read "X Setpoint (T)"() -> (w704:dbl)
        n377 = local read "Y Setpoint (T)"() -> (w703:dbl)
        n378 = local read "Z Setpoint (T)"() -> (w702:dbl)
        n379 = call-poly <vilib>:"3D Coordinate Conversion.vi"("conversion type"=w699, "axis 3"=w702, "axis 2"=w703, "axis 1"=w704) -> ("axis 3 out"=w700:dbl, "axis 2 out"=w701:dbl, "axis 1 out"=w705:dbl)  [unwired: 4 in, 1 out]
        n380 = expression code="x*180/pi"(w700) -> (w707:dbl)
        n381 = expression code="x*180/pi"(w701) -> (w706:dbl)
        n382 = local write "R Setpoint (T)"(w705) -> ()
        n383 = local write "Theta Setpoint (deg)"(w706) -> ()
        n384 = local write "Phi Setpoint (deg)"(w707) -> ()
      }
    }
    n385 = Wait (ms)(milliseconds to wait=u32 10) -> ()  [unwired: 1 out]
    n386 = local read "OK"() -> (w679:bool)
  }
  n387 = disable-structure shown="Disabled" {
    frame Disabled {
      (unwired) enum16{"write", "read"}."write" ("Function")
      (unwired) T1 "GRPX" ("Device Identifier 2")
      (unwired) FALSE
      n388 = call-poly <instrlib>:"Configuration (Read).vi"() -> ()  [unwired: 3 in, 9 out]
      n389 = local read "Magnet Response"() -> ()  [unwired: 1 in]
    }
    frame Enabled {
    }
  }
